vi "op_ACQuisition.vi"(0 "EQ folder path Refnum":refnum<vi>, 1 "HV enable button":bool caption="High Voltage enable", 2 "HV parameters Refnum":refnum<vi>, 3 "HV level Refnum":refnum<vi>, 4 "HV string Refnum":refnum<vi>, 5 "Stop ACQ button Refnum":refnum<vi>, 6 "ACQ Parameters (cluster)":T2={"Acquisition Mode"=0, "Pulse width"=0, "DTP period"=1, "Number of events"=4000} caption="Acquisition Parameters" {"Number of events" min=1; "DTP period" min=1; "Pulse width" items=["25 ns", "50 ns", "75 ns", "100 ns"]; "Acquisition Mode" items=["Normal", "Pedestal", "Test Pulse", "Test Pulse trigger & synchronous"]}, 7 "Events to acquire Refnum":refnum<vi>, 8 "error tick Refnum":refnum<vi>, 9 "ACQ events fets Refnum":refnum<vi>, 10 "Operation text Refnum":refnum<vi>, 11 "ACQ events fets A Refnum":refnum<vi>, 12 "Busy Refnum":refnum<vi>, 13 "ACQ events fets B Refnum":refnum<vi>, 14 "Addresses Cluster":T1={"ENA1"=FALSE, "IP address 1"="172.16.14.22", "ENA2"=FALSE, "IP address 2"="172.16.14.23"}, 15 "etapa# terminals refnums":T3, 17 "GbReg params":u8[](array[numeric])=[32, 22], 19 "Motors Refnum":refnum<vi>) -> (23 "Folder path: acquisition reports":path=path "C:/VIPauto/Files/LayerID/Acquisition/yyyymmdd_hh-mm-ss_Leak#_HV#")   [LabVIEW 2015, in "VIPM2.lvlib"]
uses:
  VIPM2.lvlib
panel:
  out "Chip ID list 2":u32[](array[numeric]) format="%.0x"
  out "Layer ID list 2 (ordered)":u32[](array[numeric]) format="%.0x"
  out "All ID list 2":u32[](array[numeric]) format="%.0x"
  out "All ID list 1":u32[](array[numeric]) format="%.0x"
  out "Layer ID list 1 (ordered)":u32[](array[numeric]) format="%.0x"
  out "Chip ID list 1":u32[](array[numeric]) format="%.0x"
  # "Operation: ACQuisition with HV (refnums)"
  # "Analog Vref low"
  # "Gb THLD"
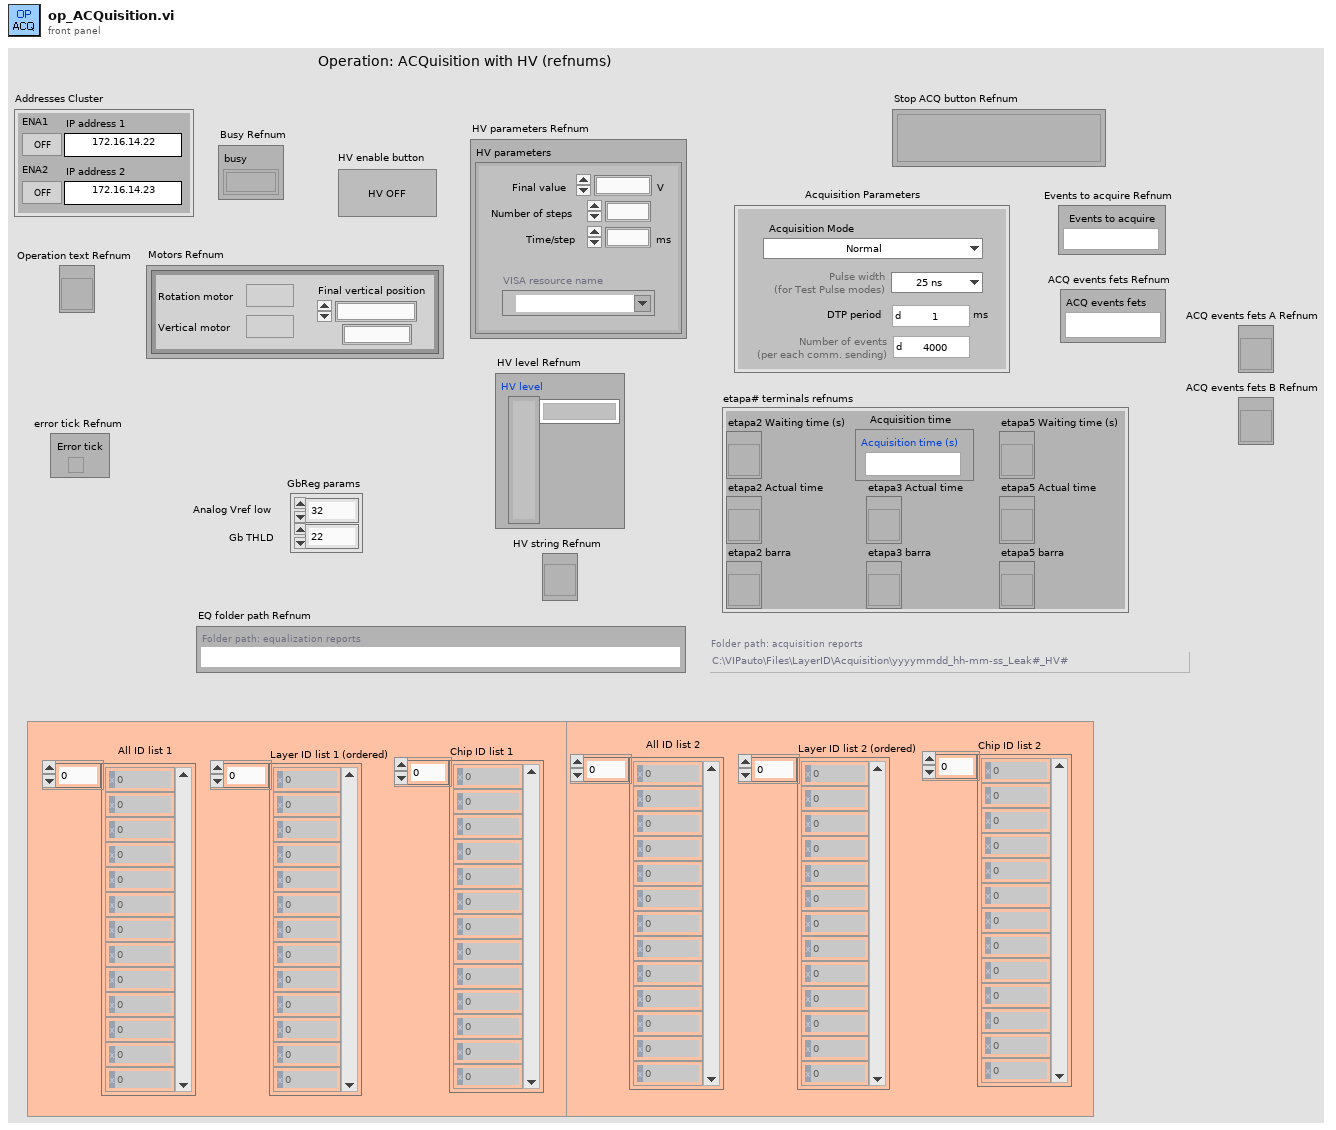
[diagram p1: front panel]
types:
  T1 = cluster{"ENA1":bool, "IP address 1":string, "ENA2":bool, "IP address 2":string}
  T2 = cluster{"Acquisition Mode":u32, "Pulse width":u32, "DTP period":u32, "Number of events":u32}
  T3 = cluster{"etapa2 Waiting time (s)":refnum<vi>, "etapa2 Actual time":refnum<vi>, "etapa2 barra":refnum<vi>, "etapa3 Actual time":refnum<vi>, "etapa3 barra":refnum<vi>, "etapa5 Waiting time (s)":refnum<vi>, "etapa5 Actual time":refnum<vi>, "etapa5 barra":refnum<vi>, "Acquisition time":refnum<vi>}
  T4 = enum8{"Enabled", "Disabled", "Disabled and Grayed Out"}
  T5 = cluster{"Final value":i16, "Number of steps":u8, "Time/step":u16, "Output Off Behavior":u16, "VISA resource name":refnum<visa-resource-name>}
  T6 = cluster{"Rotation motor":bool, "Vertical motor":bool, "Final vertical position":u32, "vertical position":u32}
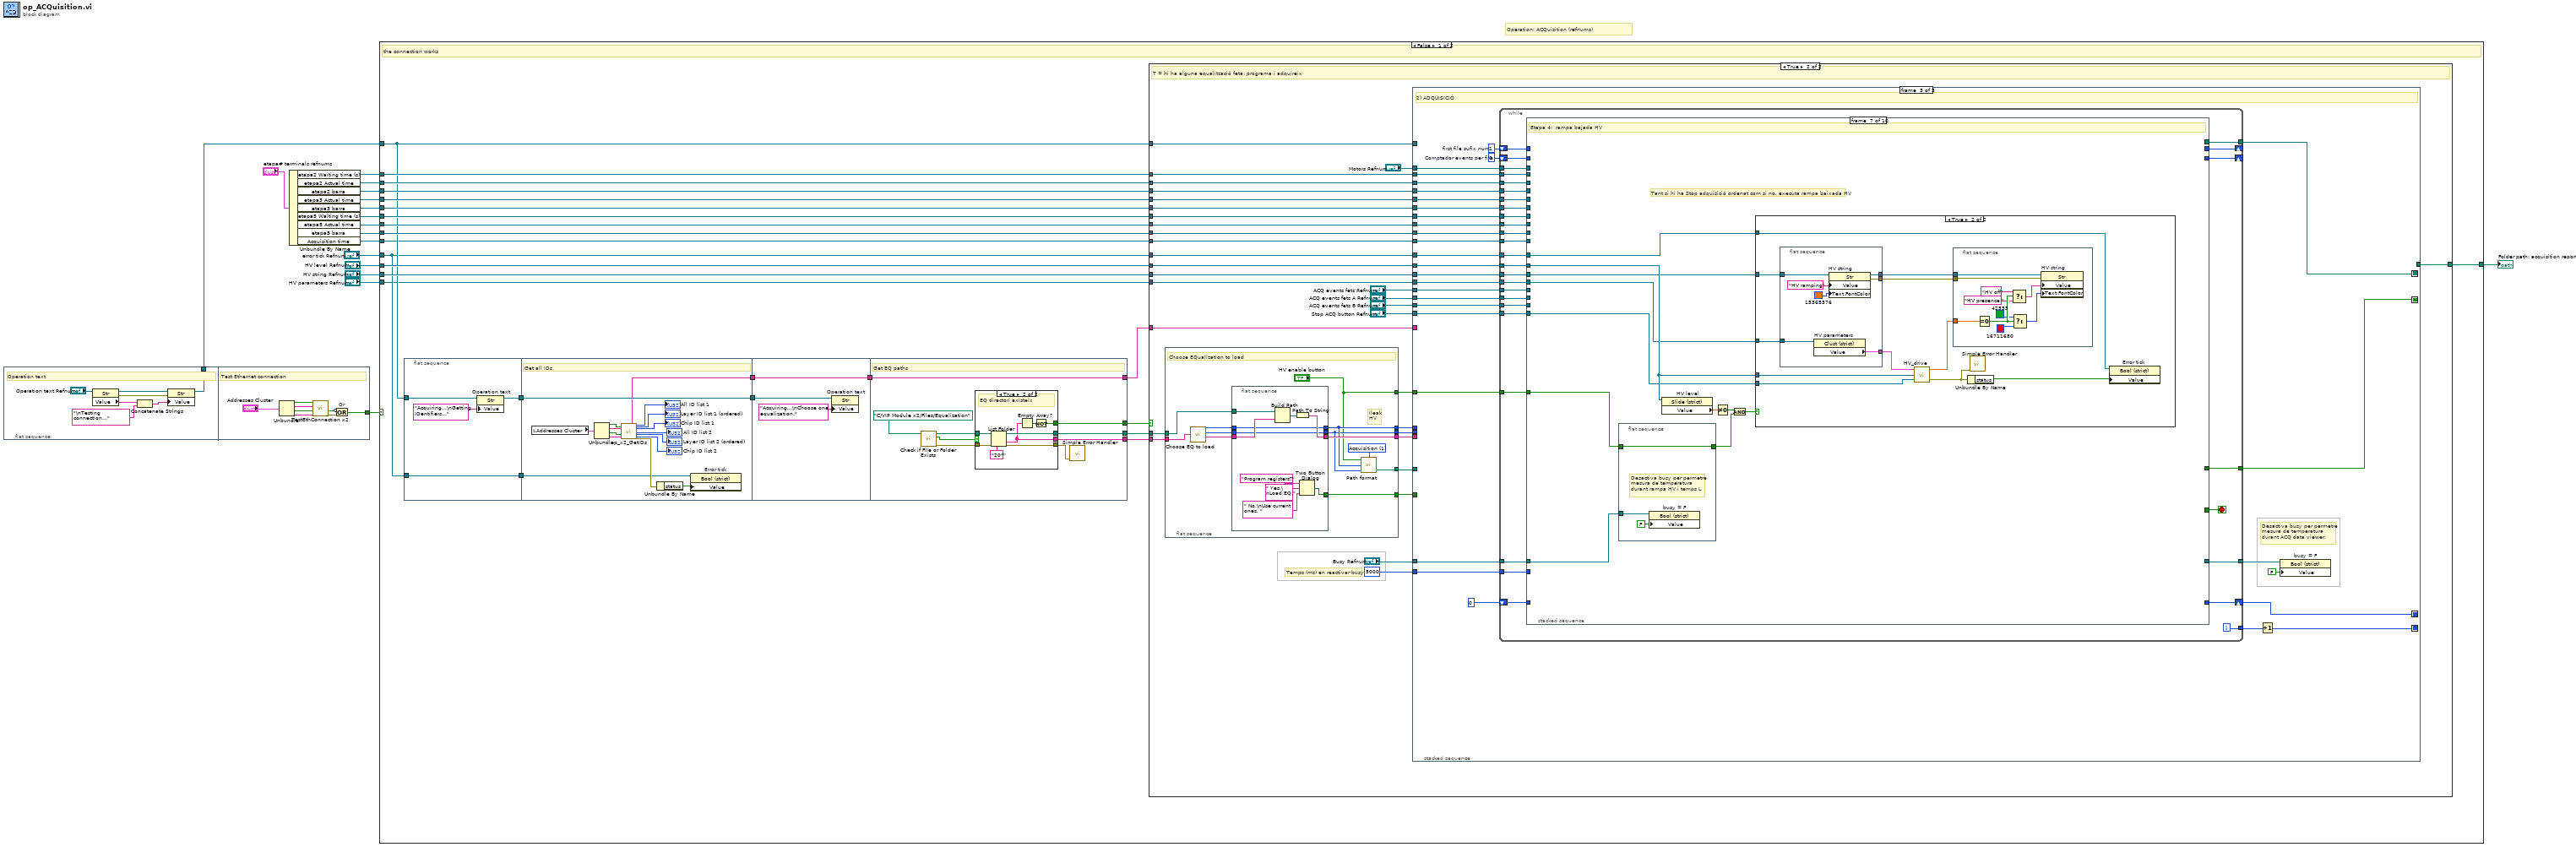
[diagram p0: block diagram]
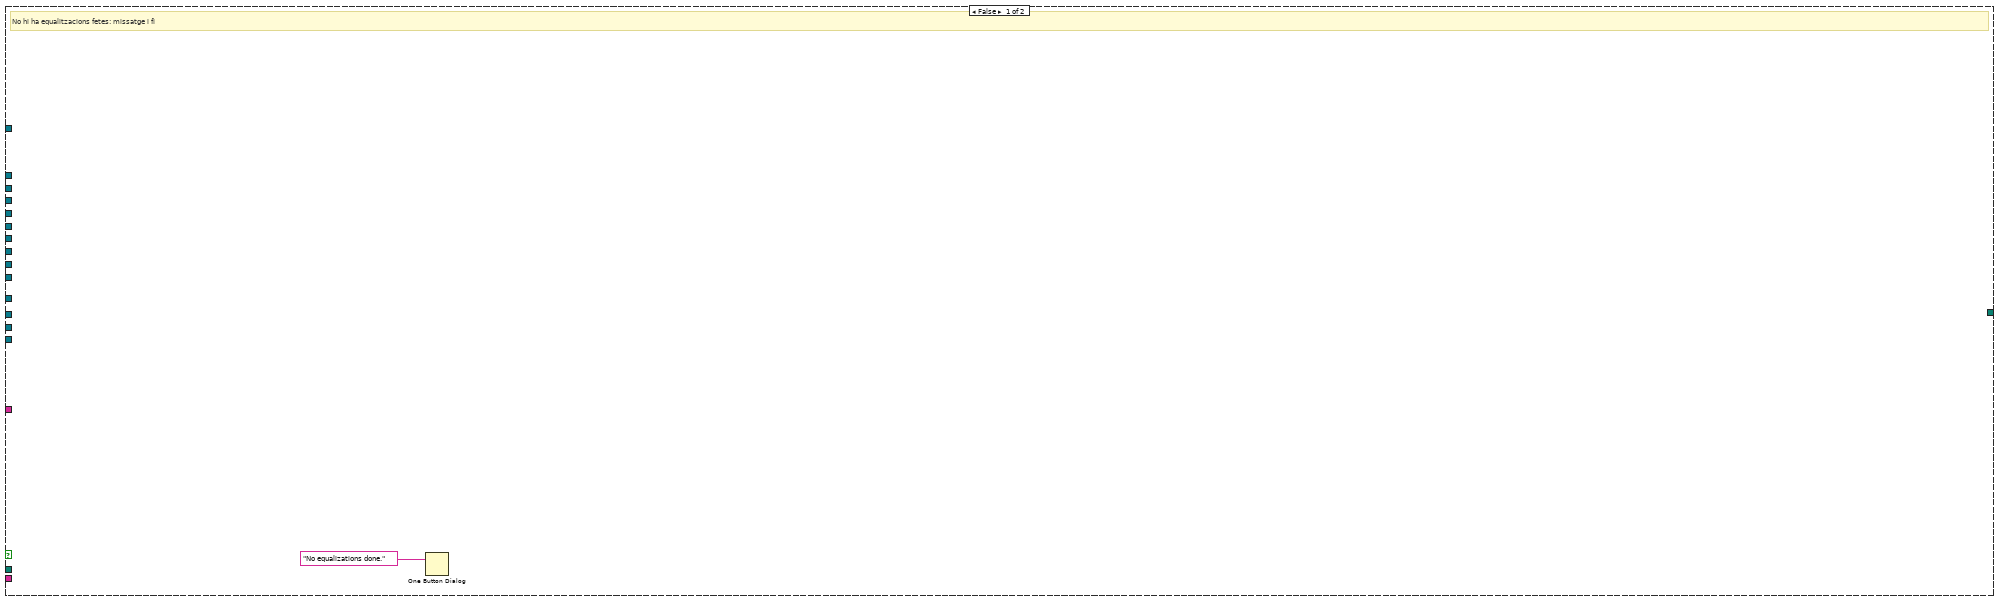
[diagram p3: hidden frame]
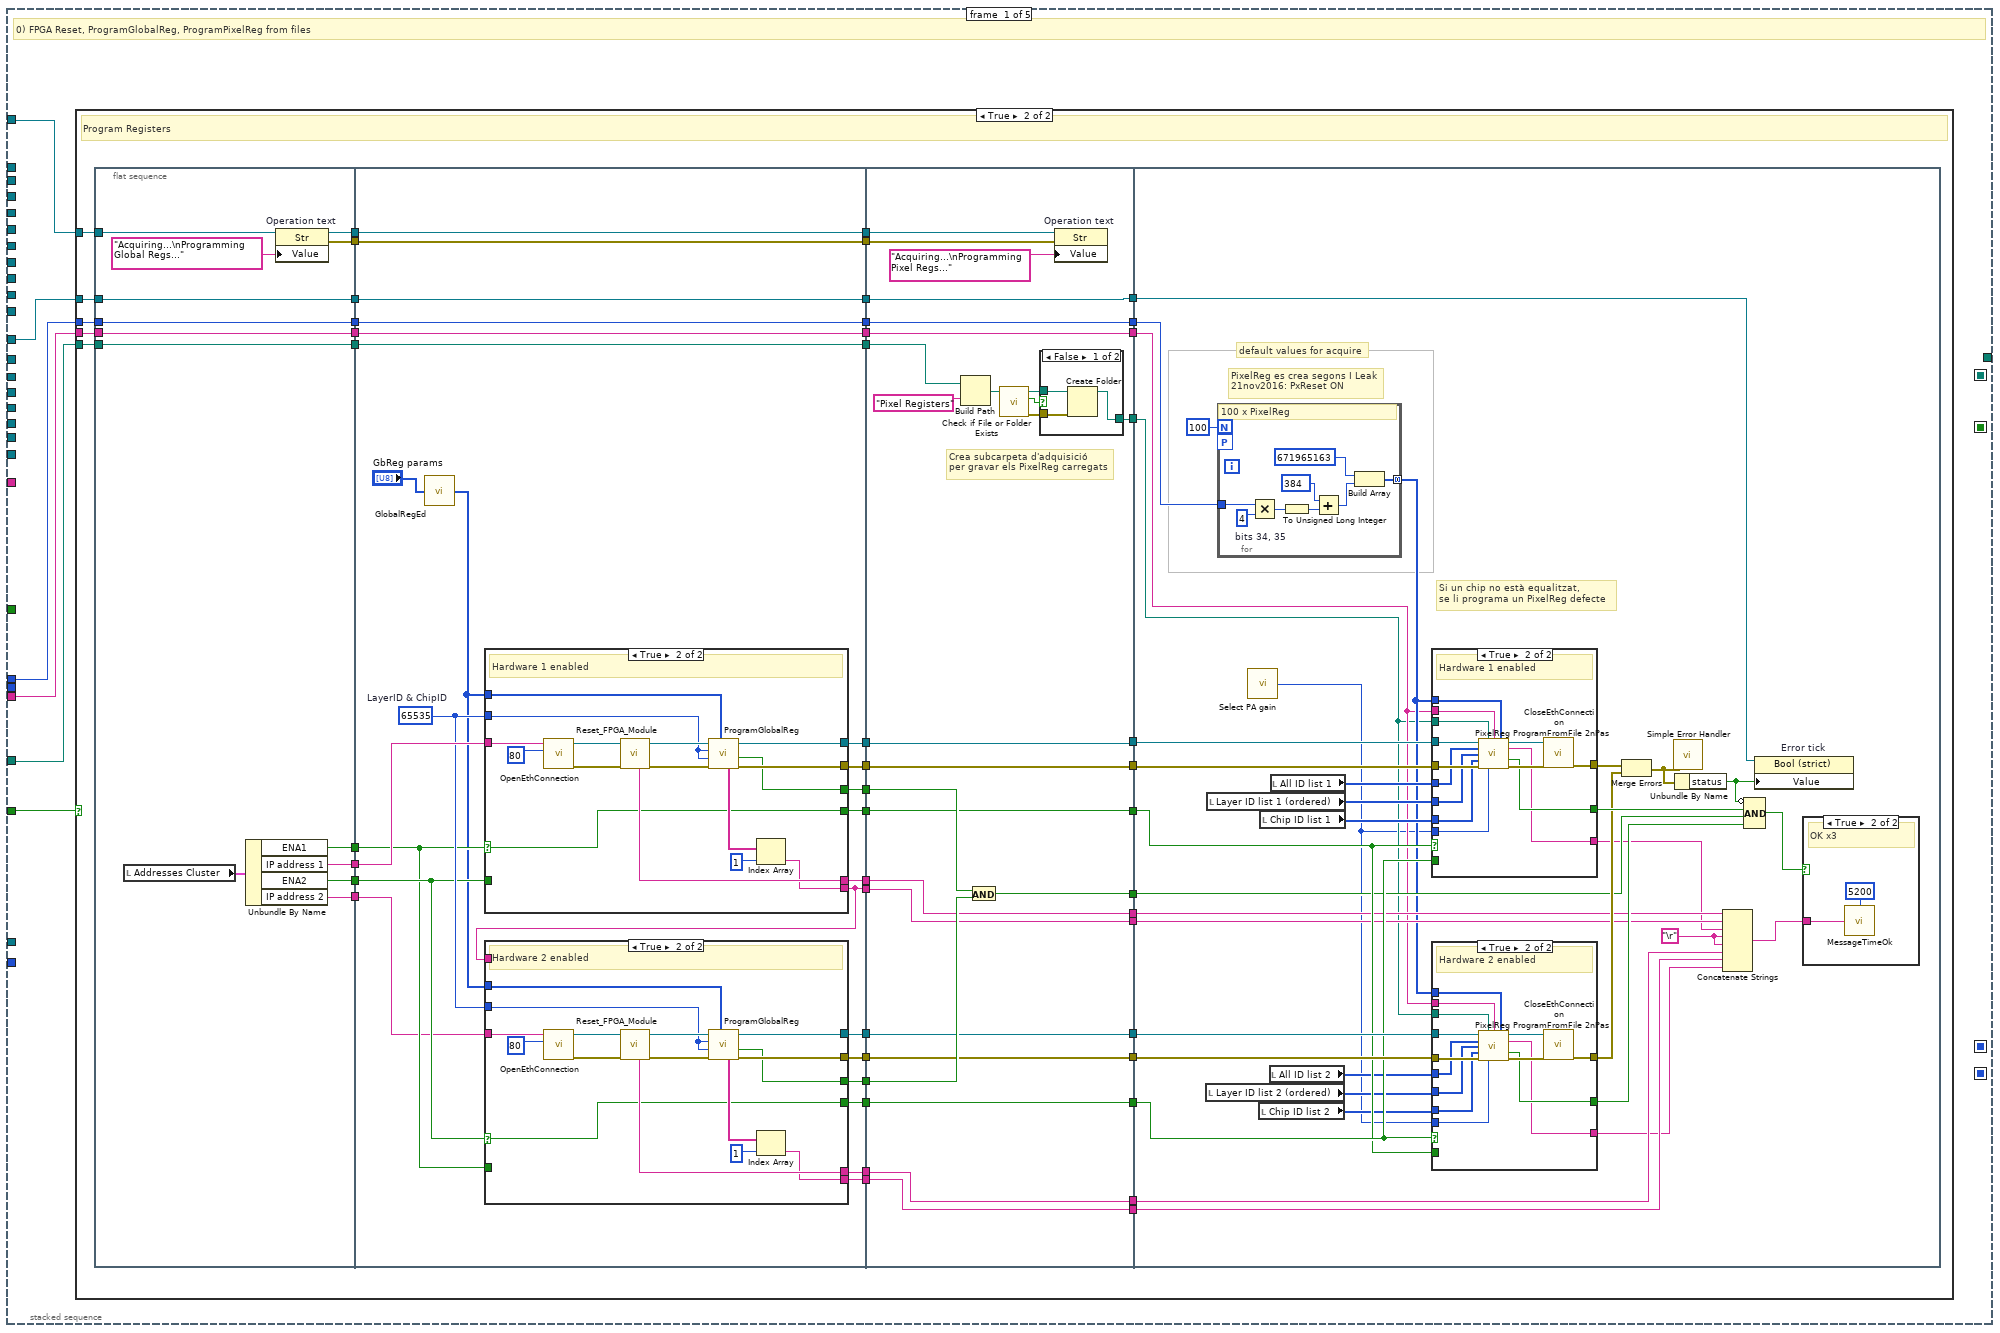
[diagram p4: hidden frame]
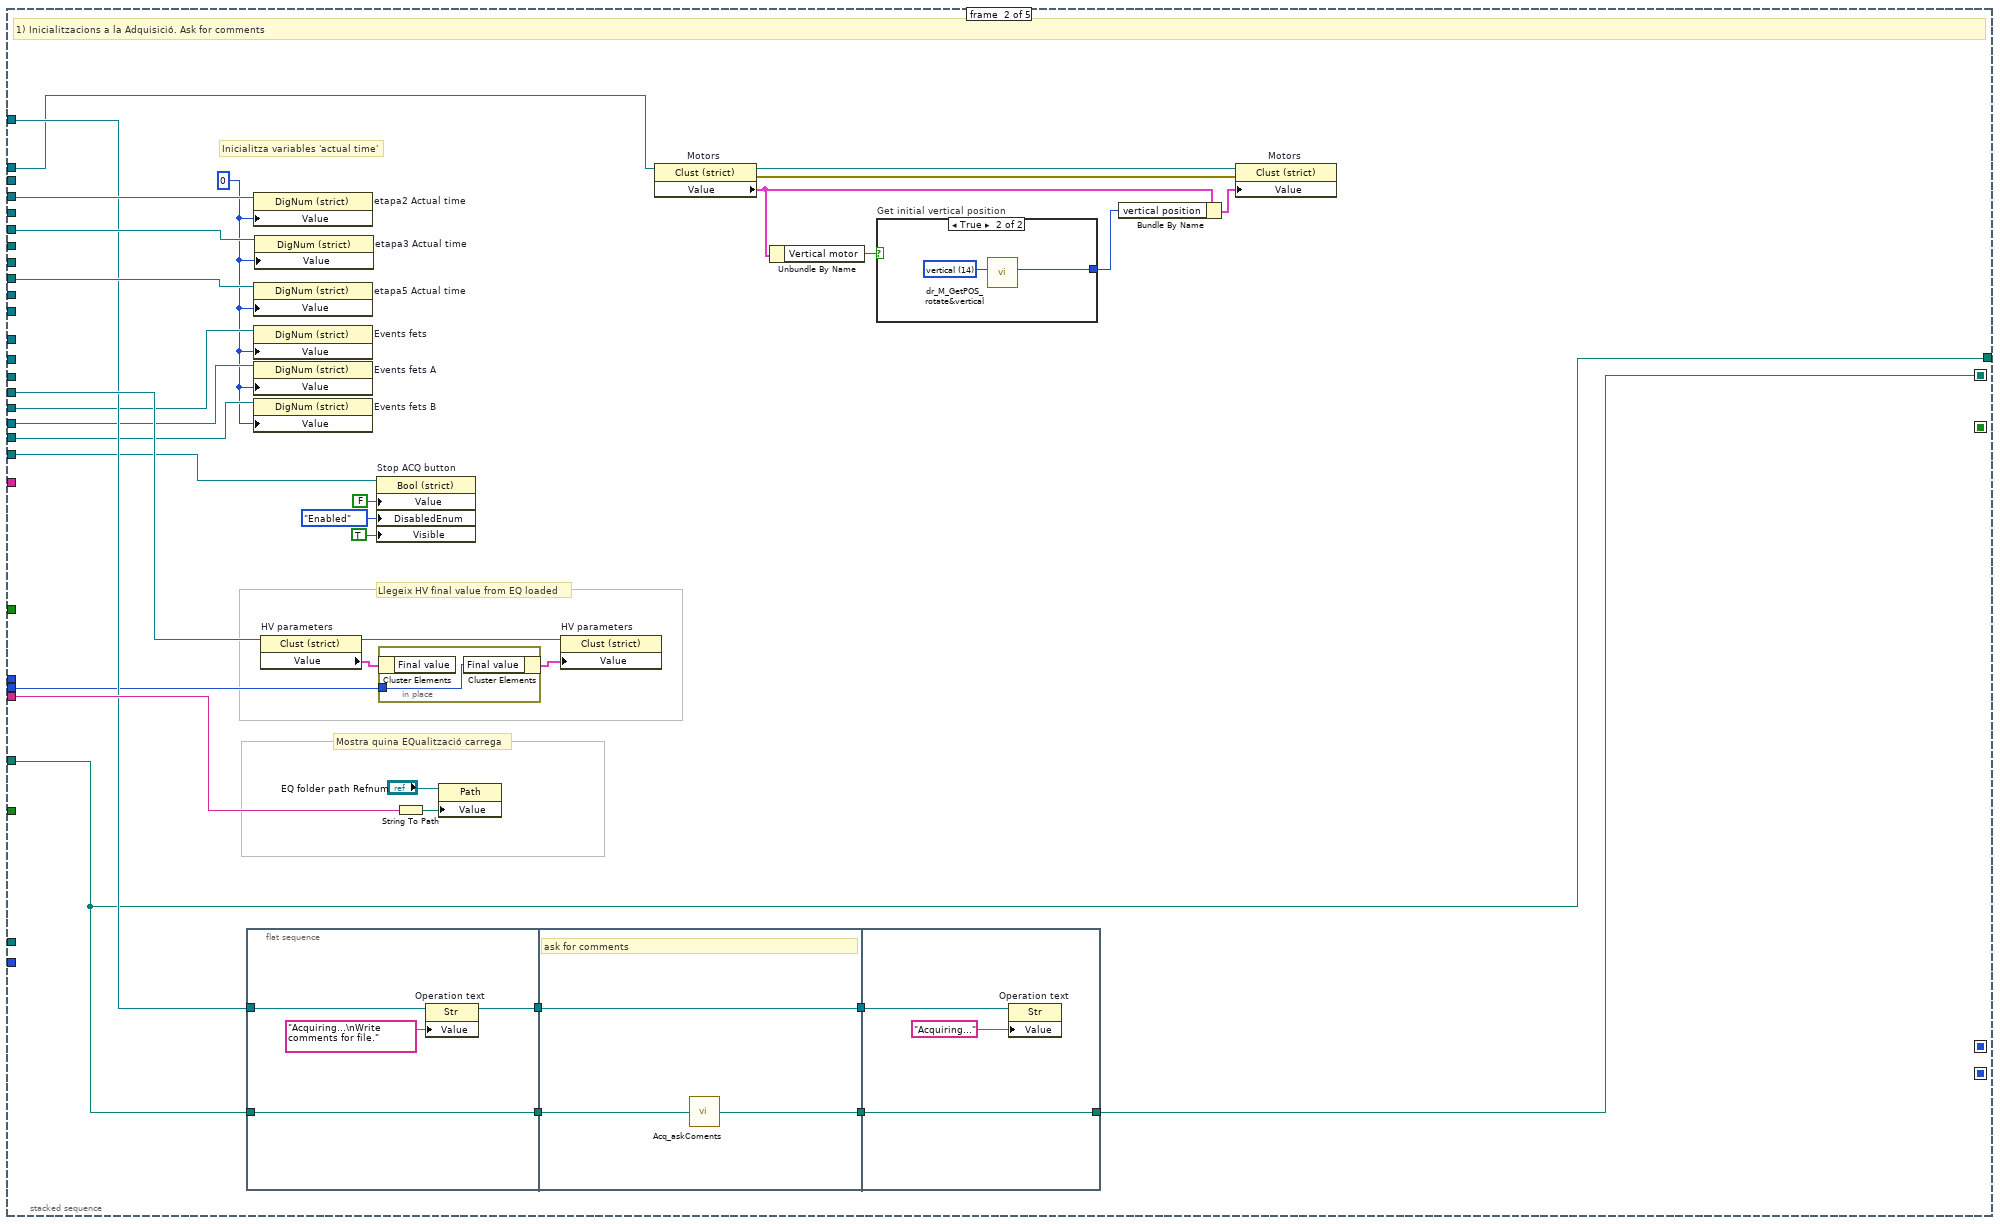
[diagram p12: hidden frame]
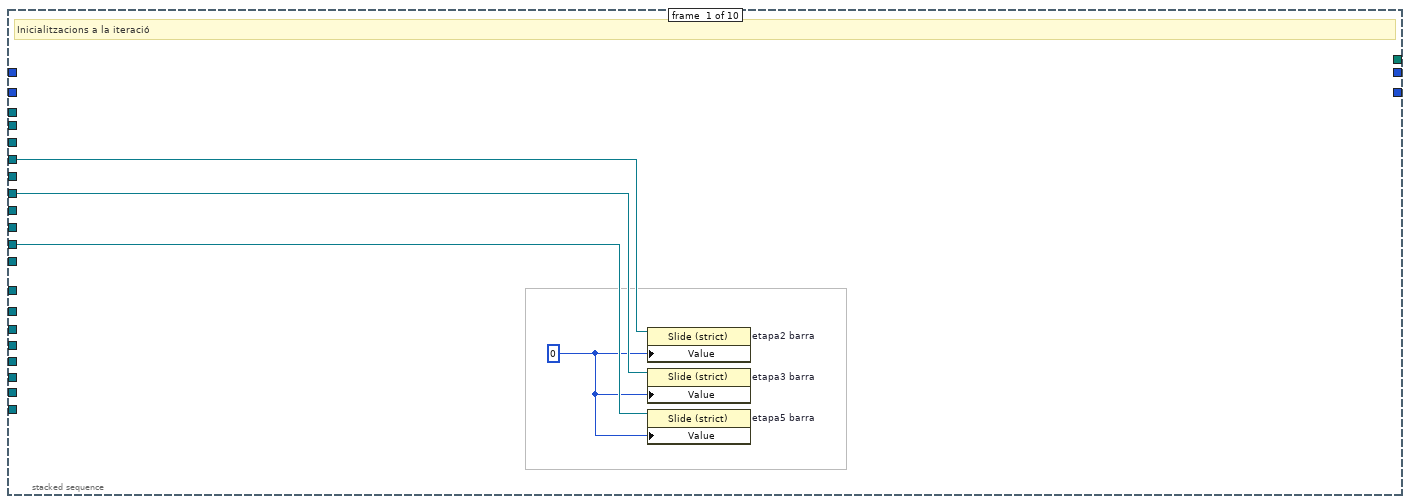
[diagram p14: hidden frame]
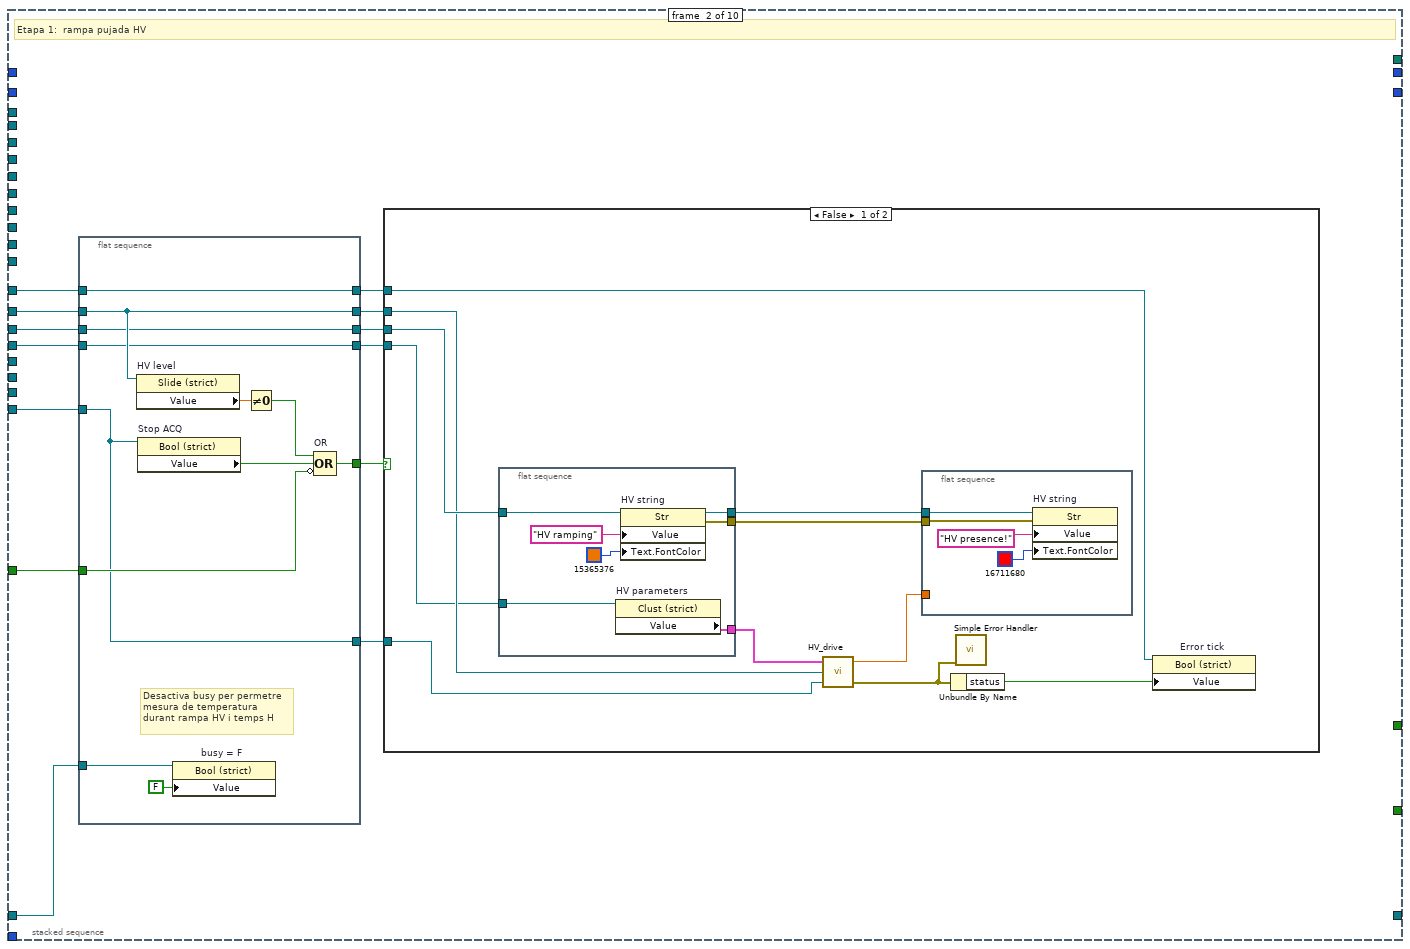
[diagram p15: hidden frame]
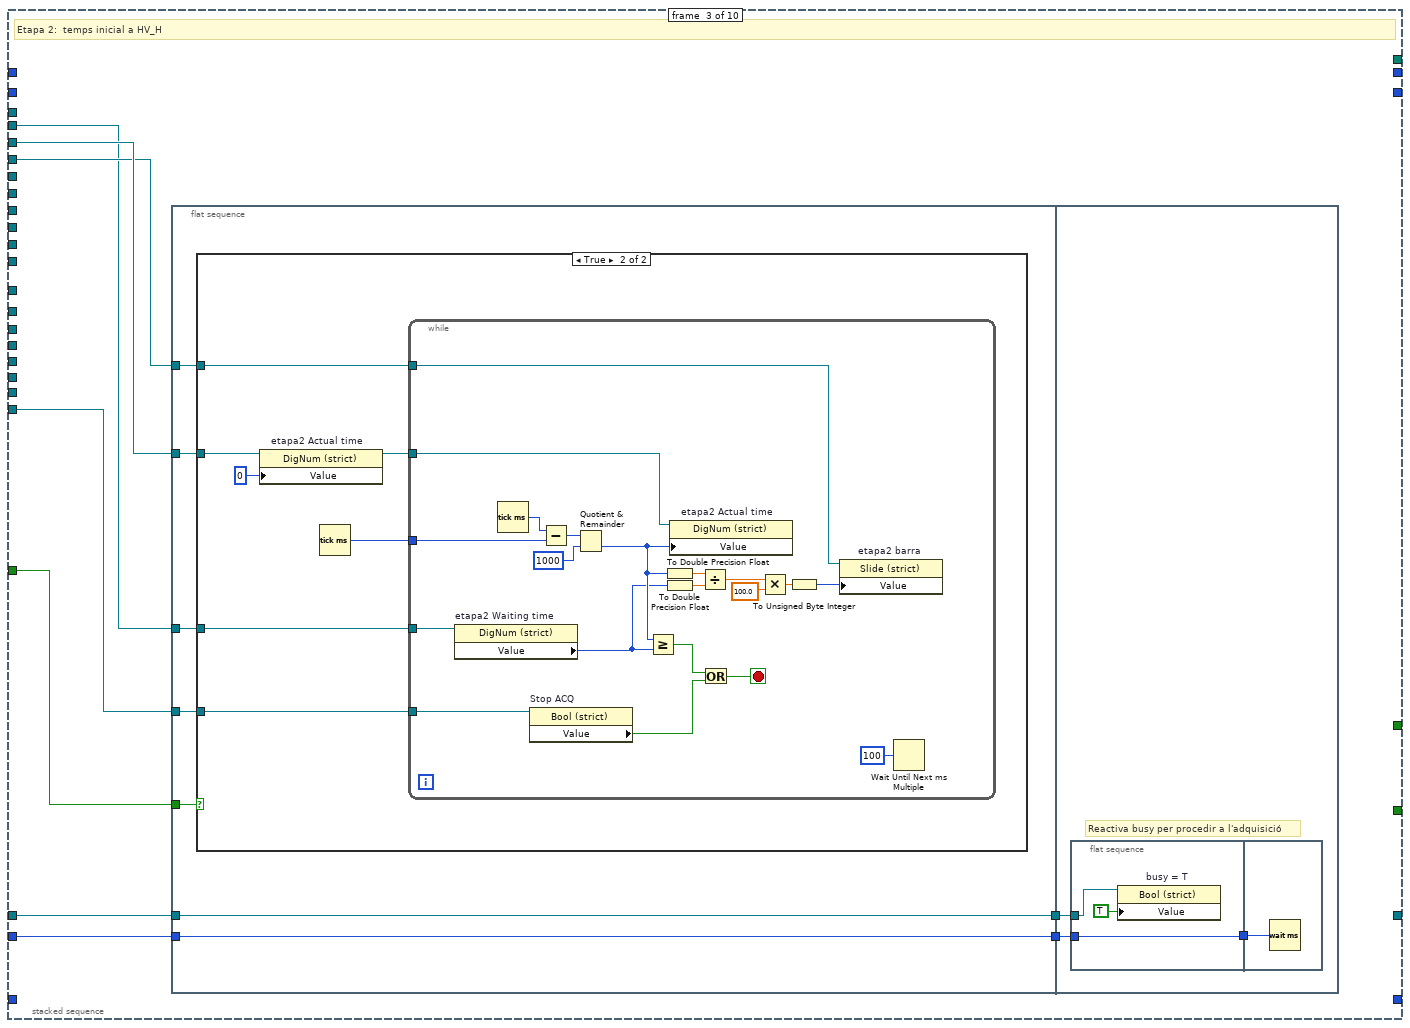
[diagram p17: hidden frame]
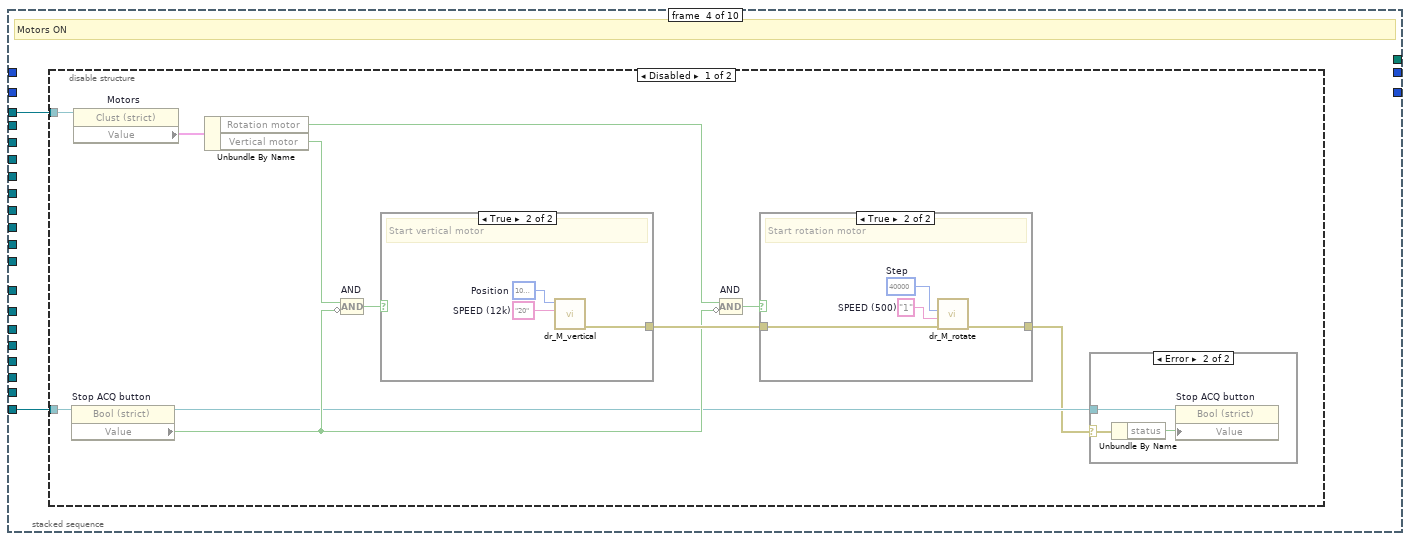
[diagram p19: hidden frame]
diagram:
  # "Operation: ACQuisition (refnums)"
  n1 = flat-sequence {
    tunnel: [w18] -> w7
    tunnel: [w30] -> w17
    frame #0 {
      # "Operation text"
      n2 = property class="Str"(reference="Operation text Refnum") -> (reference out=w21:refnum<vi>, error out=w20:errorcluster, "Value"=w23:string)  [unwired: 1 in]
      n3 = Concatenate Strings "Concatenate Strings"(w23, "\nTesting connection..." ("string")) -> (w19:string)
      n4 = property class="Str"(reference=w21, error in=w20, "Value"=w19) -> (reference out=w18:refnum<vi>)  [unwired: 1 out]
    }
    frame #1 {
      # "Test Ethernet connection"
      n5 = Unbundle("Addresses Cluster") -> ("ENA1"=w28:bool, "IP address 1"=w27:string, "ENA2"=w26:bool, "IP address 2"=w25:string)
      n6 = call "TestEthConnection x2.vi"("IP address 2"=w25, "ENA2"=w26, "IP address 1"=w27, "ENA1"=w28) -> ("error out"=w31:errorcluster, "Answers OK?"=w32:bool)  [unwired: 6 in]
      n7 = Compound Arithmetic op=OR "Or"(invert w32, w31) -> (w30:bool)
    }
  }
  n8 = Unbundle By Name("etapa# terminals refnums") -> ("etapa2 Waiting time (s)"=w15:refnum<vi>, "etapa2 Actual time"=w14:refnum<vi>, "etapa2 barra"=w13:refnum<vi>, "etapa3 Actual time"=w12:refnum<vi>, "etapa3 barra"=w11:refnum<vi>, "etapa5 Waiting time (s)"=w10:refnum<vi>, "etapa5 Actual time"=w9:refnum<vi>, "etapa5 barra"=w8:refnum<vi>, "Acquisition time"=w2:refnum<vi>)
  n9 = case shown="False" w17 {
    selector: w17 -> [_ w939]
    tunnel: w15 -> [w56 _]
    tunnel: w14 -> [w55 _]
    tunnel: w13 -> [w54 _]
    tunnel: w12 -> [w53 _]
    tunnel: w11 -> [w52 _]
    tunnel: w10 -> [w51 _]
    tunnel: w9 -> [w50 _]
    tunnel: w8 -> [w49 _]
    tunnel: w7 -> [w45 _]
    tunnel: "HV level Refnum" -> [w48 _]
    tunnel: "HV string Refnum" -> [w47 _]
    tunnel: "error tick Refnum" -> [w43 w938]
    tunnel: [w46 _] -> w1
    tunnel: "HV parameters Refnum" -> [w37 _]
    tunnel: w2 -> [w36 _]
    frame False {
      # "the connection works"
      n10 = flat-sequence {
        tunnel: w45 -> [w60]
        tunnel: [w58] -> w44
        tunnel: w43 -> [w58]
        tunnel: [w57] -> w41
        tunnel: w44 -> [w74]
        tunnel: [w73] -> w42
        tunnel: w41 -> [w73]
        tunnel: [w72] -> w34
        tunnel: w42 -> [w78]
        tunnel: [w77] -> w35
        tunnel: w34 -> [w77]
        tunnel: [w84] -> w40
        tunnel: [w83] -> w39
        tunnel: [w82] -> w38
        tunnel: [w80] -> w33
        tunnel: w35 -> [w80]
        frame #0 {
          n11 = property on="Operation text" class="Str"(reference=w60, "Value"="Acquiring...\nGetting IDentifiers...") -> (reference out=w57:refnum<vi>)  [unwired: 1 in, 1 out]
        }
        frame #1 {
          # "Get all IDs"
          n12 = local read "Addresses Cluster"() -> (w71:T1)
          n13 = Unbundle(w71) -> ("ENA1"=w70:bool, "IP address 1"=w69:string, "ENA2"=w67:bool, "IP address 2"=w68:string)
          n14 = call "op_x2_GetIDs.vi"("ENA1"=w70, "IP address 1"=w69, "ENA2"=w67, "IP address 2"=w68) -> ("summary IDs"=w72:string, "All ID list 1"=→"All ID list 1":u32[], "Layer ID list 1 (ordered)"=→"Layer ID list 1 (ordered)":u32[], "Chip ID list 1"=→"Chip ID list 1":u32[], "All ID list 2"=→"All ID list 2":u32[], "Layer ID list 2 (ordered)"=→"Layer ID list 2 (ordered)":u32[], "Chip ID list 2"=→"Chip ID list 2":u32[], "error out"=w75:errorcluster)  [unwired: 16 in]
          n15 = Unbundle By Name(w75) -> ("status"=w76:bool)
          n16 = property on="Error tick" class="Bool (strict)"(reference=w74, "Value"=w76) -> ()  [unwired: 1 in, 2 out]
        }
        frame #2 {
          n17 = property on="Operation text" class="Str"(reference=w78, "Value"="Acquiring...\nChoose one equalization.") -> ()  [unwired: 1 in, 2 out]
        }
        frame #3 {
          # "Get EQ paths"
          n18 = call <vilib>:"Check if File or Folder Exists.vi"("path"=path "C:/VIP Module x2/Files/Equalization") -> ("error out"=w85:errorcluster, "file or folder exists?"=w86:bool, "dup path"=w87:path)  [unwired: 8 in]
          n19 = case shown="True" w86 {
            selector: w86 -> [w91 _]
            tunnel: w87 -> [w90 w97]
            tunnel: w85 -> [w89 w96]
            tunnel: [w91 w93] -> w84
            tunnel: [w90 w94] -> w83
            tunnel: [w89 w95] -> w81
            tunnel: [_ w92] -> w82
            frame False {
              # "no EQs"
            }
            frame True {
              # "EQ directori existeix"
              n20 = List Folder(path=w97, pattern="20*", error in=w96) -> (path out=w94:path, folder names=w92:string[], error out=w95:errorcluster)  [unwired: 1 in, 1 out]
              n21 = Empty Array?(array=w92) -> (empty?=w98:bool)
              n22 = Not(x=w98) -> (.not. x?=w93:bool)
            }
          }
          n23 = call <vilib>:"Simple Error Handler.vi"("error in (no error)"=w81) -> ()  [unwired: 4 in, 5 out]
        }
      }
      n24 = case shown="True" w40 {
        tunnel: w56 -> [_ w131]
        tunnel: w55 -> [_ w130]
        tunnel: w54 -> [_ w129]
        tunnel: w53 -> [_ w128]
        tunnel: w52 -> [_ w127]
        tunnel: w51 -> [_ w126]
        tunnel: w50 -> [_ w125]
        tunnel: w49 -> [_ w124]
        tunnel: w48 -> [_ w123]
        tunnel: w47 -> [_ w122]
        tunnel: [_ w121] -> w46
        tunnel: w45 -> [_ w120]
        tunnel: w43 -> [_ w119]
        tunnel: w39 -> [_ w118]
        tunnel: w38 -> [_ w117]
        tunnel: w37 -> [_ w113]
        tunnel: w36 -> [_ w110]
        tunnel: w33 -> [_ w108]
        frame False {
          # "No hi ha equalitzacions fetes: missatge i fi"
          n25 = One Button Dialog(message="No equalizations done.") -> ()  [unwired: 1 in, 1 out]
        }
        frame True {
          # "Temps (ms) en reactivar busy"
          # "T = hi ha alguna equalització feta: programa i adquireix"
          n26 = flat-sequence {
            tunnel: w118 -> [w140]
            tunnel: w117 -> [w141]
            tunnel: [w138] -> w116
            tunnel: [w133] -> w115
            tunnel: [w136] -> w114
            tunnel: [w142] -> w112
            tunnel: [w137] -> w107
            tunnel: ["HV enable button"] -> w104
            frame #0 {
              w143 = u8 1 items=["Equalization", "Acquisition"] ("Operation type")
              # "Ileak\nHV"
              # "Choose EQualization to load"
              n27 = call "Choose EQ to load.vi"("EQ folders"=w141) -> ("I Leakage"=w135:u8, "HV last value"=w134:i16, "loaded EQ folder"=w139:string)  [unwired: 5 in]
              n28 = flat-sequence {
                tunnel: w140 -> [w153]
                tunnel: w139 -> [w152]
                tunnel: [w150] -> w138
                tunnel: [w149] -> w137
                tunnel: [w145] -> w136
                tunnel: w135 -> [w145]
                tunnel: w134 -> [w144]
                tunnel: [w144] -> w133
                frame #0 {
                  n29 = Build Path(base path=w153, name or relative path=w152) -> (appended path=w151:path)
                  n30 = Path To String(path=w151) -> (string=w150:string)
                  n31 = Two Button Dialog(message="Program registers?", 1:" No.\nUse current ones. " ("F button name (\"Cancel\")"), 2:" Yes.\nLoad EQ." ("T button name (\"OK\")")) -> (T button?=w149:bool)
                }
              }
              n32 = call "Path format.vi"("Operation type"=w143, "HV level"=w133, "I leakage"=w136, "HV enable button"="HV enable button") -> ("folder path"=w142:path)  [unwired: 1 in]
            }
          }
          n33 = stacked-sequence {
            seq-local: [_ _ w450 _ _] -> [_ _ _ _ w890]
            seq-local: [_ w406 _ _ _] -> [_ _ w451 _ w889]
            seq-local: [_ _ w441 _ _] -> [_ _ _ _ w868]
            seq-local: [_ _ w439 _ _] -> [_ _ _ _ w867]
            tunnel: w120 -> [w159 w411 _ _ w887]
            tunnel: w131 -> [_ _ w465 _ w874]
            tunnel: w130 -> [_ w421 w464 _ _]
            tunnel: w129 -> [_ _ w463 _ _]
            tunnel: w128 -> [_ w420 w462 _ _]
            tunnel: w127 -> [_ _ w461 _ _]
            tunnel: w126 -> [_ _ w460 _ w876]
            tunnel: w125 -> [_ w419 w459 _ _]
            tunnel: w124 -> [_ _ w458 _ _]
            tunnel: w119 -> [w158 _ w455 _ _]
            tunnel: w123 -> [_ _ w457 _ _]
            tunnel: w122 -> [_ _ w456 _ _]
            tunnel: [_ w404 _ _ _] -> w121
            tunnel: w116 -> [w157 w412 _ _ w881]
            tunnel: w115 -> [_ w410 _ _ _]
            tunnel: w114 -> [w156 _ _ _ _]
            tunnel: w113 -> [_ w418 w454 _ w885]
            tunnel: w112 -> [w155 w404 _ _ w882]
            tunnel: "Stop ACQ button Refnum" -> [_ w403 w453 w866 _]
            tunnel: w110 -> [_ _ w452 _ w875]
            tunnel: "ACQ events fets Refnum" -> [_ w399 w449 _ w880]
            tunnel: w108 -> [_ _ _ _ w888]
            tunnel: w107 -> [w154 _ _ _ w883]
            tunnel: "Busy Refnum" -> [_ _ w448 _ _]
            tunnel: u32 5000 -> [_ _ w447 _ _]
            tunnel: w104 -> [_ _ w443 _ _]
            tunnel: "ACQ events fets A Refnum" -> [_ w398 w438 _ _]
            tunnel: "ACQ events fets B Refnum" -> [_ w397 w437 _ _]
            tunnel: "Motors Refnum" -> [_ w395 w435 _ _]
            frame #0 {
              # "0) FPGA Reset, ProgramGlobalReg, ProgramPixelReg from files"
              n34 = case shown="True" w154 {
                tunnel: w159 -> [_ w190]
                tunnel: w158 -> [_ w189]
                tunnel: w157 -> [_ w188]
                tunnel: w156 -> [_ w187]
                tunnel: w155 -> [_ w186]
                frame False {
                  # "Use current registers values"
                }
                frame True {
                  # "Program Registers"
                  n35 = flat-sequence {
                    tunnel: w190 -> [w219]
                    tunnel: [w218] -> w207
                    tunnel: [w217] -> w206
                    tunnel: [w216] -> w205
                    tunnel: w189 -> [w216]
                    tunnel: [w215] -> w204
                    tunnel: w188 -> [w215]
                    tunnel: [w214] -> w203
                    tunnel: w187 -> [w214]
                    tunnel: [w213] -> w202
                    tunnel: w186 -> [w213]
                    tunnel: [w211] -> w185
                    tunnel: [w210] -> w184
                    tunnel: [w209] -> w183
                    tunnel: [w208] -> w182
                    tunnel: w207 -> [w245]
                    tunnel: w206 -> [w244]
                    tunnel: [w245] -> w201
                    tunnel: [w244] -> w200
                    tunnel: [w243] -> w199
                    tunnel: w205 -> [w243]
                    tunnel: w204 -> [w242]
                    tunnel: [w242] -> w198
                    tunnel: w203 -> [w241]
                    tunnel: [w241] -> w197
                    tunnel: w202 -> [w240]
                    tunnel: [w240] -> w196
                    tunnel: w185 -> [w236]
                    tunnel: w184 -> [w237]
                    tunnel: w183 -> [w239]
                    tunnel: w182 -> [w235]
                    tunnel: [w234] -> w181
                    tunnel: [w233] -> w180
                    tunnel: [w232] -> w179
                    tunnel: [w231] -> w178
                    tunnel: [w230] -> w177
                    tunnel: [w223] -> w176
                    tunnel: [w229] -> w175
                    tunnel: [w228] -> w174
                    tunnel: [w227] -> w173
                    tunnel: [w226] -> w172
                    tunnel: [w225] -> w171
                    tunnel: [w224] -> w170
                    tunnel: w201 -> [w306]
                    tunnel: w200 -> [w305]
                    tunnel: [w292] -> w195
                    tunnel: [w291] -> w194
                    tunnel: [w304] -> w193
                    tunnel: w199 -> [w304]
                    tunnel: [w303] -> w192
                    tunnel: w198 -> [w303]
                    tunnel: [w302] -> w191
                    tunnel: w197 -> [w302]
                    tunnel: w196 -> [w294]
                    tunnel: w181 -> [w292]
                    tunnel: w180 -> [w291]
                    tunnel: w179 -> [w301]
                    tunnel: w178 -> [w290]
                    tunnel: w177 -> [w285]
                    tunnel: w176 -> [w284]
                    tunnel: w175 -> [w289]
                    tunnel: w174 -> [w288]
                    tunnel: w173 -> [w300]
                    tunnel: w172 -> [w287]
                    tunnel: w171 -> [w283]
                    tunnel: w170 -> [w282]
                    tunnel: [w293] -> w169
                    tunnel: [w290] -> w168
                    tunnel: [w289] -> w167
                    tunnel: [w288] -> w166
                    tunnel: [w287] -> w165
                    tunnel: [w286] -> w164
                    tunnel: [w285] -> w163
                    tunnel: [w284] -> w162
                    tunnel: [w283] -> w161
                    tunnel: [w282] -> w160
                    tunnel: w195 -> [w341]
                    tunnel: w194 -> [w340]
                    tunnel: w193 -> [w343]
                    tunnel: w192 -> [w319]
                    tunnel: w191 -> [w338]
                    tunnel: w169 -> [w318]
                    tunnel: w168 -> [w331]
                    tunnel: w167 -> [w334]
                    tunnel: w166 -> [w333]
                    tunnel: w165 -> [w332]
                    tunnel: w164 -> [w324]
                    tunnel: w163 -> [w322]
                    tunnel: w162 -> [w321]
                    tunnel: w161 -> [w315]
                    tunnel: w160 -> [w314]
                    frame #0 {
                      n36 = local read "Addresses Cluster"() -> (w212:T1)
                      n37 = Unbundle By Name(w212) -> ("ENA1"=w211:bool, "IP address 1"=w209:string, "ENA2"=w210:bool, "IP address 2"=w208:string)
                      n38 = property on="Operation text" class="Str"(reference=w219, "Value"="Acquiring...\nProgramming Global Regs...") -> (reference out=w218:refnum<vi>, error out=w217:errorcluster)  [unwired: 1 in]
                    }
                    frame #1 {
                      w238 = u32 65535  # LayerID & ChipID
                      n39 = call "GlobalRegEd.vi"("params"="GbReg params") -> ("Global Reg out"=w222:u32[])  [unwired: 4 in]
                      n40 = case shown="True" w236 {
                        selector: w236 -> [w265 w266]
                        tunnel: w238 -> [_ w268]
                        tunnel: [_ w274] -> w234
                        tunnel: [_ w273] -> w233
                        tunnel: [_ w272] -> w230
                        tunnel: [_ w271] -> w223
                        tunnel: [w264 w270] -> w232
                        tunnel: w222 -> [_ w269]
                        tunnel: w239 -> [_ w267]
                        tunnel: [w265 w266] -> w231
                        tunnel: w237 -> [w264 _]
                        frame False {
                          # "Hardware 1 not enabled"
                        }
                        frame True {
                          # "Hardware 1 enabled"
                          n41 = call "OpenEthConnection.vi"("Port"=u16 80, "IP address"=w267) -> ("error out"=w280:errorcluster, "connection ID out"=w281:refnum<k5>)  [unwired: 7 in, 1 out]
                          n42 = call "Reset_FPGA_Module.vi"("error in (no error)"=w280, "connection ID"=w281) -> ("error out"=w277:errorcluster, "connection ID out"=w278:refnum<k5>, "Answer to Reset"=w272:string)  [unwired: 7 in]
                          n43 = call "ProgramGlobalReg.vi"("Global Reg"=w269, "error in (no error)"=w277, "ChipID"=w268, "LayerID"=w268, "connection ID"=w278) -> ("error out"=w273:errorcluster, "OK?"=w270:bool, "connection ID out"=w274:refnum<k5>, "Program done"=w276:string[])  [unwired: 2 in, 1 out]
                          n44 = Index Array "Index Array"(array=w276, index=1) -> (element=w271:string)
                        }
                      }
                      n45 = case shown="True" w237 {
                        selector: w237 -> [w247 w248]
                        tunnel: w238 -> [_ w250]
                        tunnel: [_ w256] -> w229
                        tunnel: [_ w255] -> w228
                        tunnel: [_ w254] -> w225
                        tunnel: [_ w253] -> w224
                        tunnel: [w246 w252] -> w227
                        tunnel: w222 -> [_ w251]
                        tunnel: w235 -> [_ w249]
                        tunnel: [w247 w248] -> w226
                        tunnel: w236 -> [w246 _]
                        tunnel: w223 -> [_ _]
                        frame False {
                          # "Hardware 2 not enabled"
                        }
                        frame True {
                          # "Hardware 2 enabled"
                          n46 = call "OpenEthConnection.vi"("Port"=u16 80, "IP address"=w249) -> ("error out"=w262:errorcluster, "connection ID out"=w263:refnum<k5>)  [unwired: 7 in, 1 out]
                          n47 = call "Reset_FPGA_Module.vi"("error in (no error)"=w262, "connection ID"=w263) -> ("error out"=w259:errorcluster, "connection ID out"=w260:refnum<k5>, "Answer to Reset"=w254:string)  [unwired: 7 in]
                          n48 = call "ProgramGlobalReg.vi"("Global Reg"=w251, "error in (no error)"=w259, "ChipID"=w250, "LayerID"=w250, "connection ID"=w260) -> ("error out"=w255:errorcluster, "OK?"=w252:bool, "connection ID out"=w256:refnum<k5>, "Program done"=w258:string[])  [unwired: 2 in, 1 out]
                          n49 = Index Array "Index Array"(array=w258, index=1) -> (element=w253:string)
                        }
                      }
                    }
                    frame #2 {
                      # "Crea subcarpeta d'adquisició\nper gravar els PixelReg carregats"
                      n50 = Build Path(base path=w294, name or relative path="Pixel Registers") -> (appended path=w298:path)
                      n51 = And(x=w301, y=w300) -> (x .and. y?=w286:bool)
                      n52 = call <vilib>:"Check if File or Folder Exists.vi"("path"=w298) -> ("error out"=w295:errorcluster, "file or folder exists?"=w297:bool, "dup path"=w296:path)  [unwired: 8 in]
                      n53 = case shown="False" w297 {
                        tunnel: w296 -> [w310 w311]
                        tunnel: w295 -> [w309 _]
                        tunnel: [w308 w311] -> w293
                        frame False {
                          n54 = Create Folder(path (use dialog)=w310, error in=w309) -> (created path=w308:path)  [unwired: 1 in, 2 out]
                        }
                        frame True {
                        }
                      }
                      n55 = property on="Operation text" class="Str"(reference=w306, error in=w305, "Value"="Acquiring...\nProgramming Pixel Regs...") -> ()  [unwired: 2 out]
                    }
                    frame #3 {
                      w316 = "\r"
                      # "Si un chip no està equalitzat,\nse li programa un PixelReg defecte"
                      # "default values for acquire"
                      # "PixelReg es crea segons I Leak\n21nov2016: PxReset ON"
                      n56 = local read "Layer ID list 2 (ordered)"() -> (w329:u32[])
                      n57 = local read "Layer ID list 1 (ordered)"() -> (w336:u32[])
                      n58 = for {
                        N: 100 -> [_]
                        tunnel: w338 -> [w382]
                        tunnel: [w379] -> w320 mode=concatenating
                        workers-P: _ -> [_]
                        w386 = u8 4  # bits 34, 35
                        # "100 x PixelReg"
                        n59 = Multiply(x=w382, y=w386) -> (x*y=w384:u8)
                        n60 = To Unsigned Long Integer(number=w384) -> (unsigned 32bit integer=w383:u32)
                        n61 = Add(x=u32 384, y=w383) -> (x+y=w380:u32)
                        n62 = Build Array(u32 671965163 ("Numeric"), w380) -> (w379:u32[])
                      }
                      n63 = call "Select PA gain.vi"() -> ("PA gain selected"=w312:u8)  [unwired: 5 in]
                      n64 = local read "Chip ID list 2"() -> (w328:u32[])
                      n65 = local read "Chip ID list 1"() -> (w335:u32[])
                      n66 = local read "All ID list 2"() -> (w330:u32[])
                      n67 = local read "All ID list 1"() -> (w337:u32[])
                      n68 = case shown="True" w331 {
                        tunnel: [w364 w378] -> w326
                        tunnel: w341 -> [_ w377]
                        tunnel: w340 -> [w364 w376]
                        tunnel: [w363 w373] -> w339
                        tunnel: w320 -> [_ w372]
                        tunnel: w319 -> [_ w371]
                        tunnel: w318 -> [_ w370]
                        tunnel: [_ w369] -> w317
                        tunnel: w337 -> [_ w366]
                        tunnel: w336 -> [_ w367]
                        tunnel: w335 -> [_ w368]
                        tunnel: w332 -> [w363 _]
                        tunnel: w312 -> [_ w365]
                        frame False {
                          # "Hardware 1 not enabled"
                        }
                        frame True {
                          # "Hardware 1 enabled"
                          n69 = call "PixelReg ProgramFromFile 2nPas.vi"("connection ID"=w377, "ACQ PxReg folder"=w370, "EQ folder path"=w371, "PixelReg (hex)"=w372, "All ID list"=w366, "Layer ID list"=w367, "Chip ID list"=w368, "error in (no error)"=w376, "PA gain"=w365) -> ("connection ID out"=w375:refnum<k5>, "done message"=w369:string, "All checks OK"=w373:bool, "error out (no error)"=w374:errorcluster)  [unwired: 2 in, 1 out]
                          n70 = call "CloseEthConnection.vi"("error in (no error)"=w374, "connection ID"=w375) -> ("error out"=w378:errorcluster)  [unwired: 9 in]
                        }
                      }
                      n71 = case shown="True" w332 {
                        tunnel: [w348 w362] -> w325
                        tunnel: w334 -> [_ w361]
                        tunnel: w333 -> [w348 w360]
                        tunnel: [w347 w357] -> w323
                        tunnel: w320 -> [_ w356]
                        tunnel: w319 -> [_ w355]
                        tunnel: w318 -> [_ w354]
                        tunnel: [_ w353] -> w313
                        tunnel: w330 -> [_ w350]
                        tunnel: w329 -> [_ w351]
                        tunnel: w328 -> [_ w352]
                        tunnel: w331 -> [w347 _]
                        tunnel: w312 -> [_ w349]
                        frame False {
                          # "Hardware 2 not enabled"
                        }
                        frame True {
                          # "Hardware 2 enabled"
                          n72 = call "PixelReg ProgramFromFile 2nPas.vi"("connection ID"=w361, "ACQ PxReg folder"=w354, "EQ folder path"=w355, "PixelReg (hex)"=w356, "All ID list"=w350, "Layer ID list"=w351, "Chip ID list"=w352, "error in (no error)"=w360, "PA gain"=w349) -> ("connection ID out"=w359:refnum<k5>, "done message"=w353:string, "All checks OK"=w357:bool, "error out (no error)"=w358:errorcluster)  [unwired: 2 in, 1 out]
                          n73 = call "CloseEthConnection.vi"("error in (no error)"=w358, "connection ID"=w359) -> ("error out"=w362:errorcluster)  [unwired: 9 in]
                        }
                      }
                      n74 = Merge Errors(w326, w325) -> (w327:errorcluster)
                      n75 = call <vilib>:"Simple Error Handler.vi"("error in (no error)"=w327) -> ()  [unwired: 4 in, 5 out]
                      n76 = Unbundle By Name(w327) -> ("status"=w342:bool)
                      n77 = Concatenate Strings "Concatenate Strings"(w322, w321, w317, w316, w316, w315, w314, w313) -> (w345:string)
                      n78 = Compound Arithmetic op=AND(invert w342, w339, w324, w323) -> (w344:bool)
                      n79 = property on="Error tick" class="Bool (strict)"(reference=w343, "Value"=w342) -> ()  [unwired: 1 in, 2 out]
                      n80 = case shown="True" w344 {
                        tunnel: w345 -> [_ w388]
                        frame False {
                          # "error"
                        }
                        frame True {
                          # "OK x3"
                          n81 = call "MessageTimeOk.vi"("time (ms)"=5200, "missage"=w388) -> ()  [unwired: 4 in]
                        }
                      }
                    }
                  }
                }
              }
            }
            frame #1 {
              w396 = u32 0 ("Value")
              # "Mostra quina EQualització carrega"
              # "Llegeix HV final value from EQ loaded"
              # "Inicialitza variables 'actual time'"
              # "1) Inicialitzacions a la Adquisició. Ask for comments"
              n82 = flat-sequence {
                tunnel: w411 -> [w426]
                tunnel: [w425] -> w407
                tunnel: [w424] -> w405
                tunnel: w404 -> [w424]
                tunnel: [w430] -> w409
                tunnel: [w429] -> w408
                tunnel: w407 -> [w429]
                tunnel: w405 -> [w428]
                tunnel: [w433] -> w406
                tunnel: w409 -> [w433]
                tunnel: w408 -> [w432]
                frame #0 {
                  n83 = property on="Operation text" class="Str"(reference=w426, "Value"="Acquiring...\nWrite comments for file.") -> (reference out=w425:refnum<vi>)  [unwired: 1 in, 1 out]
                }
                frame #1 {
                  # "ask for comments"
                  n84 = call "Acq_askComents.vi"("Folder path"=w428) -> ("Complete file path"=w430:path)  [unwired: 4 in]
                }
                frame #2 {
                  n85 = property on="Operation text" class="Str"(reference=w432, "Value"="Acquiring...") -> ()  [unwired: 1 in, 2 out]
                }
              }
              n86 = property on="etapa2 Actual time" class="DigNum (strict)"(reference=w421, "Value"=w396) -> ()  [unwired: 1 in, 2 out]
              n87 = property on="etapa5 Actual time" class="DigNum (strict)"(reference=w419, "Value"=w396) -> ()  [unwired: 1 in, 2 out]
              n88 = property on="Events fets" class="DigNum (strict)"(reference=w399, "Value"=w396) -> ()  [unwired: 1 in, 2 out]
              n89 = property on="Events fets A" class="DigNum (strict)"(reference=w398, "Value"=w396) -> ()  [unwired: 1 in, 2 out]
              n90 = property on="Events fets B" class="DigNum (strict)"(reference=w397, "Value"=w396) -> ()  [unwired: 1 in, 2 out]
              n91 = property on="etapa3 Actual time" class="DigNum (strict)"(reference=w420, "Value"=w396) -> ()  [unwired: 1 in, 2 out]
              n92 = property on="HV parameters" class="Clust (strict)"(reference=w418) -> (reference out=w415:refnum<vi>, "Value"=w417:T5)  [unwired: 1 in, 1 out]
              n93 = property on="Stop ACQ button" class="Bool (strict)"(reference=w403, "Value"=FALSE, "DisabledEnum"=T4."Enabled" ("Disabled"), "Visible"=TRUE) -> ()  [unwired: 1 in, 2 out]
              n94 = in-place {
                in-place-border: w410 -> [w434]
                n95 = in-place-cluster #1(w417) -> ()  [unwired: 1 out]
                n96 = in-place-cluster #1("Final value"=w434) -> (w416:T5)
              }
              n97 = String To Path(string=w412) -> (path=w413:path)
              n98 = property class="Path"(reference="EQ folder path Refnum", "Value"=w413) -> ()  [unwired: 1 in, 2 out]
              n99 = property on="HV parameters" class="Clust (strict)"(reference=w415, "Value"=w416) -> ()  [unwired: 1 in, 2 out]
              n100 = property on="Motors" class="Clust (strict)"(reference=w395) -> (reference out=w393:refnum<vi>, error out=w392:errorcluster, "Value"=w391:T6)  [unwired: 1 in]
              n101 = Unbundle By Name(w391) -> ("Vertical motor"=w394:bool)
              n102 = case "Get initial vertical position" shown="True" w394 {
                tunnel: [_ w422] -> w390
                frame False {
                }
                frame True {
                  w423 = u8 14 items=["rotating"=6, "vertical"=14] ("motor")
                  n103 = call "dr_M_GetPOS_rotate&vertical.vi"("motor"=w423) -> ("POSition"=w422:u32)  [unwired: 9 in, 1 out]
                }
              }
              n104 = Bundle By Name(cluster=w391, "vertical position"=w390) -> (w389:T6)
              n105 = property on="Motors" class="Clust (strict)"(reference=w393, error in=w392, "Value"=w389) -> ()  [unwired: 2 out]
            }
            frame #2 {
              w436 = u32 0  # Comptador events per file
              w444 = u32 1  # first file sufix num.
              # "Desactiva busy per permetre\nmesura de temperatura\ndurant ACQ data viewer."
              # "2) ADQUISICIÓ"
              n106 = while {
                tunnel: w465 -> [w497]
                tunnel: w464 -> [w496]
                tunnel: w463 -> [w495]
                tunnel: w462 -> [w494]
                tunnel: w461 -> [w493]
                tunnel: w460 -> [w492]
                tunnel: w459 -> [w491]
                tunnel: w458 -> [w490]
                tunnel: w457 -> [w489]
                tunnel: w456 -> [w488]
                tunnel: w455 -> [w487]
                tunnel: w454 -> [w486]
                tunnel: w453 -> [w485]
                tunnel: w443 -> [w484]
                tunnel: w452 -> [w483]
                tunnel: w451 -> [w482]
                tunnel: [w481] -> w450
                tunnel: w449 -> [w479]
                tunnel: w448 -> [w478]
                tunnel: w447 -> [w477]
                tunnel: [w476] -> w445
                shift-right: [w474] -> _
                shift-left: w444 -> [w475]
                tunnel: [w473] -> w442
                shift-right: [w471] -> w439
                shift-left: u32 0 -> [w472]
                tunnel: w438 -> [w470]
                tunnel: w437 -> [w469]
                shift-right: [w467] -> _
                shift-left: w436 -> [w468]
                tunnel: w435 -> [w466]
                i -> [w473]
                stop <- w480 stop-if-true
                n107 = stacked-sequence {
                  tunnel: w497 -> [_ _ w555 _ _ _ _ _ _ _]
                  tunnel: w496 -> [_ _ w557 _ _ _ _ _ _ _]
                  tunnel: w495 -> [w501 _ w556 _ _ _ _ _ _ _]
                  tunnel: w494 -> [_ _ _ _ w632 _ _ _ _ w860]
                  tunnel: w493 -> [w500 _ _ _ w631 _ _ _ _ _]
                  tunnel: w492 -> [_ _ _ _ _ _ _ _ w806 _]
                  tunnel: w491 -> [_ _ _ _ _ _ _ _ w807 _]
                  tunnel: w490 -> [w499 _ _ _ _ _ _ _ w805 _]
                  tunnel: w489 -> [_ w513 _ _ _ _ w723 _ _ _]
                  tunnel: w488 -> [_ w506 _ _ _ _ w722 _ _ _]
                  tunnel: w487 -> [_ w509 _ _ w634 _ w721 _ _ _]
                  tunnel: w486 -> [_ w504 _ _ _ _ w720 _ _ _]
                  tunnel: w485 -> [_ w514 w554 w600 w630 w682 w714 w756 w804 w863]
                  tunnel: w484 -> [_ w511 w553 _ _ _ w717 _ w803 _]
                  tunnel: w483 -> [_ _ _ _ w636 _ _ _ _ _]
                  tunnel: w482 -> [_ _ _ _ w635 _ _ _ w798 _]
                  tunnel: [_ _ _ _ w633 _ _ _ _ _] -> w481
                  tunnel: [_ _ _ _ _ _ _ _ _ w862] -> w480
                  tunnel: w479 -> [_ _ _ _ w628 _ _ _ _ _]
                  tunnel: w478 -> [_ w503 w551 _ w624 _ w715 _ w801 w861]
                  tunnel: w477 -> [_ _ w549 _ _ _ _ _ w799 _]
                  tunnel: [_ _ _ _ _ _ _ _ _ w861] -> w476
                  tunnel: w475 -> [_ _ _ _ _ _ _ _ w790 _]
                  tunnel: [_ _ _ _ _ _ _ _ w797 _] -> w474
                  tunnel: w472 -> [_ _ _ _ _ _ _ _ _ w859]
                  tunnel: [_ _ _ _ _ _ _ _ _ w857] -> w471
                  tunnel: w470 -> [_ _ _ _ w627 _ _ _ _ _]
                  tunnel: w469 -> [_ _ _ _ w626 _ _ _ _ _]
                  tunnel: w468 -> [_ _ _ _ _ _ _ _ w791 _]
                  tunnel: [_ _ _ _ _ _ _ _ w796 _] -> w467
                  tunnel: w466 -> [_ _ _ w599 _ w683 _ w757 _ _]
                  frame #0 {
                    w498 = u8 0 ("ACQ-e2 barra")
                    # "Inicialitzacions a la iteració"
                    n108 = property on="etapa2 barra" class="Slide (strict)"(reference=w501, "Value"=w498) -> ()  [unwired: 1 in, 2 out]
                    n109 = property on="etapa3 barra" class="Slide (strict)"(reference=w500, "Value"=w498) -> ()  [unwired: 1 in, 2 out]
                    n110 = property on="etapa5 barra" class="Slide (strict)"(reference=w499, "Value"=w498) -> ()  [unwired: 1 in, 2 out]
                  }
                  frame #1 {
                    # "Etapa 1:  rampa pujada HV"
                    n111 = flat-sequence {
                      tunnel: w514 -> [w515]
                      tunnel: w513 -> [w520]
                      tunnel: [w523] -> w512
                      tunnel: w511 -> [w522]
                      tunnel: [w521] -> w510
                      tunnel: w509 -> [w521]
                      tunnel: [w520] -> w508
                      tunnel: [w519] -> w507
                      tunnel: w506 -> [w519]
                      tunnel: [w518] -> w505
                      tunnel: w504 -> [w518]
                      tunnel: w503 -> [w516]
                      tunnel: [w515] -> w502
                      frame #0 {
                        # "Desactiva busy per permetre\nmesura de temperatura\ndurant rampa HV i temps H"
                        n112 = property on="HV level" class="Slide (strict)"(reference=w520) -> ("Value"=w526:dbl)  [unwired: 1 in, 2 out]
                        n113 = property on="Stop ACQ" class="Bool (strict)"(reference=w515) -> ("Value"=w524:bool)  [unwired: 1 in, 2 out]
                        n114 = property on="busy = F" class="Bool (strict)"(reference=w516, "Value"=FALSE) -> ()  [unwired: 1 in, 2 out]
                        n115 = Not Equal To 0?(x=w526) -> (x != 0?=w525:bool)
                        n116 = Compound Arithmetic op=OR "OR"(w525, w524, invert w522) -> (w523:bool)
                      }
                    }
                    n117 = case shown="False" w512 {
                      tunnel: w507 -> [w534 _]
                      tunnel: w508 -> [w531 _]
                      tunnel: w510 -> [w530 _]
                      tunnel: w505 -> [w528 _]
                      tunnel: w502 -> [w527 _]
                      frame False {
                        n118 = flat-sequence {
                          tunnel: [w543] -> w537
                          tunnel: w534 -> [w548]
                          tunnel: [w546] -> w533
                          tunnel: [w545] -> w532
                          tunnel: w528 -> [w542]
                          frame #0 {
                            n119 = property on="HV parameters" class="Clust (strict)"(reference=w542) -> ("Value"=w543:T5)  [unwired: 1 in, 2 out]
                            n120 = property on="HV string" class="Str"(reference=w548, "Value"="HV ramping" ("HV String"), "Text.FontColor"=u32 15365376) -> (reference out=w546:refnum<vi>, error out=w545:errorcluster)  [unwired: 1 in]
                          }
                        }
                        n121 = call "HV_drive.vi"("Stop subVI Refnum"=w527, "HV level Refnum"=w531, "HV parameters"=w537) -> ("error out"=w536:errorcluster, "HV level (last value)"=w535:dbl)  [unwired: 1 in]
                        n122 = flat-sequence {
                          tunnel: w535 -> [_]
                          tunnel: w533 -> [w540]
                          tunnel: w532 -> [w539]
                          frame #0 {
                            n123 = property on="HV string" class="Str"(reference=w540, error in=w539, "Value"="HV presence!" ("HV String"), "Text.FontColor"=u32 16711680) -> ()  [unwired: 2 out]
                          }
                        }
                        n124 = Unbundle By Name(w536) -> ("status"=w529:bool)
                        n125 = call <vilib>:"Simple Error Handler.vi"("error in (no error)"=w536) -> ()  [unwired: 4 in, 5 out]
                        n126 = property on="Error tick" class="Bool (strict)"(reference=w530, "Value"=w529) -> ()  [unwired: 1 in, 2 out]
                      }
                      frame True {
                        # "executant aturada\no hi ha HV manual\no HV not enabled"
                      }
                    }
                  }
                  frame #2 {
                    # "Etapa 2:  temps inicial a HV_H"
                    n127 = flat-sequence {
                      tunnel: w557 -> [w564]
                      tunnel: w556 -> [w563]
                      tunnel: w555 -> [w562]
                      tunnel: w554 -> [w561]
                      tunnel: w553 -> [w560]
                      tunnel: [w559] -> w552
                      tunnel: w551 -> [w559]
                      tunnel: [w558] -> w550
                      tunnel: w549 -> [w558]
                      tunnel: w552 -> [w593]
                      tunnel: w550 -> [w592]
                      frame #0 {
                        n128 = case shown="True" w560 {
                          tunnel: w564 -> [_ w570]
                          tunnel: w563 -> [_ w568]
                          tunnel: w562 -> [_ w567]
                          tunnel: w561 -> [_ w566]
                          frame False {
                          }
                          frame True {
                            n129 = property on="etapa2 Actual time" class="DigNum (strict)"(reference=w570, "Value"=u32 0 ("ACQ-e2 Actual time")) -> (reference out=w569:refnum<vi>)  [unwired: 1 in, 1 out]
                            n130 = Tick Count (ms)() -> (millisecond timer value=w571:u32)
                            n131 = while {
                              tunnel: w571 -> [w590]
                              tunnel: w569 -> [w580]
                              tunnel: w567 -> [w579]
                              tunnel: w568 -> [w577]
                              tunnel: w566 -> [w573]
                              stop <- w575 stop-if-true
                              n132 = property on="etapa2 Waiting time" class="DigNum (strict)"(reference=w579) -> ("Value"=w578:u32)  [unwired: 1 in, 2 out]
                              n133 = Tick Count (ms)() -> (millisecond timer value=w591:u32)
                              n134 = property on="Stop ACQ" class="Bool (strict)"(reference=w573) -> ("Value"=w572:bool)  [unwired: 1 in, 2 out]
                              n135 = Subtract(x=w591, y=w590) -> (x-y=w589:u32)
                              n136 = Quotient & Remainder(x=w589, y=u32 1000) -> (floor(x/y)=w581:u32)  [unwired: 1 out]
                              n137 = Greater Or Equal?(x=w581, y=w578) -> (x >= y?=w574:bool)
                              n138 = To Double Precision Float(number=w581) -> (double precision float=w582:dbl)
                              n139 = To Double Precision Float(number=w578) -> (double precision float=w583:dbl)
                              n140 = property on="etapa2 Actual time" class="DigNum (strict)"(reference=w580, "Value"=w581) -> ()  [unwired: 1 in, 2 out]
                              n141 = Divide(x=w582, y=w583) -> (x/y=w586:dbl)
                              n142 = Or(x=w574, y=w572) -> (x .or. y?=w575:bool)
                              n143 = Multiply(x=w586, y=100.0) -> (x*y=w584:dbl)
                              n144 = To Unsigned Byte Integer(number=w584) -> (unsigned 8bit integer=w576:u8)
                              n145 = property on="etapa2 barra" class="Slide (strict)"(reference=w577, "Value"=w576) -> ()  [unwired: 1 in, 2 out]
                              n146 = Wait Until Next ms Multiple(millisecond multiple=u32 100) -> ()  [unwired: 1 out]
                            }
                          }
                        }
                      }
                      frame #1 {
                        # "Reactiva busy per procedir a l'adquisició"
                        n147 = flat-sequence {
                          tunnel: w593 -> [w597]
                          tunnel: w592 -> [w595]
                          tunnel: [w595] -> w594
                          tunnel: w594 -> [w598]
                          frame #0 {
                            n148 = property on="busy = T" class="Bool (strict)"(reference=w597, "Value"=TRUE) -> ()  [unwired: 1 in, 2 out]
                          }
                          frame #1 {
                            n149 = Wait (ms)(milliseconds to wait=w598) -> ()  [unwired: 1 out]
                          }
                        }
                      }
                    }
                  }
                  frame #3 {
                    # "Motors ON"
                    n150 = disable-structure shown="Disabled" {
                      disable-tunnel: w600 -> [w611 _]
                      disable-tunnel: w599 -> [w610 _]
                      frame Disabled {
                        n151 = property on="Stop ACQ button" class="Bool (strict)"(reference=w611) -> (reference out=w602:refnum<vi>, "Value"=w603:bool)  [unwired: 1 in, 1 out]
                        n152 = property on="Motors" class="Clust (strict)"(reference=w610) -> ("Value"=w609:T6)  [unwired: 1 in, 2 out]
                        n153 = Unbundle By Name(w609) -> ("Rotation motor"=w605:bool, "Vertical motor"=w608:bool)
                        n154 = Compound Arithmetic op=AND "AND"(w608, invert w603) -> (w607:bool)
                        n155 = case shown="True" w607 {
                          tunnel: [_ w620] -> w604
                          frame False {
                          }
                          frame True {
                            w621 = "20"  # SPEED (12k)
                            w622 = 1000000  # Position
                            # "Start vertical motor"
                            n156 = call "dr_M_vertical.vi"("SPEED (12k)"=w621, "Position"=w622) -> ("error out"=w620:errorcluster)  [unwired: 9 in]
                          }
                        }
                        n157 = Compound Arithmetic op=AND "AND"(w605, invert w603) -> (w606:bool)
                        n158 = case shown="True" w606 {
                          tunnel: w604 -> [w615 w619]
                          tunnel: [w615 w618] -> w601
                          frame False {
                          }
                          frame True {
                            w616 = "1"  # SPEED (500)
                            w617 = 40000  # Step
                            # "Start rotation motor"
                            n159 = call "dr_M_rotate.vi"("error in"=w619, "SPEED (500)"=w616, "movement"=w617) -> ("error out"=w618:errorcluster)  [unwired: 8 in]
                          }
                        }
                        n160 = case shown="Error" w601 {
                          selector: w601 -> [_ w613]
                          tunnel: w602 -> [_ w614]
                          frame No Error {
                          }
                          frame Error {
                            n161 = Unbundle By Name(w613) -> ("status"=w612:bool)
                            n162 = property on="Stop ACQ button" class="Bool (strict)"(reference=w614, "Value"=w612) -> ()  [unwired: 1 in, 2 out]
                          }
                        }
                      }
                      frame Enabled {
                      }
                    }
                  }
                  frame #4 {
                    # "Etapa 3:  adquisició"
                    n163 = property on="Stop ACQ button" class="Bool (strict)"(reference=w630) -> ("Value"=w629:bool)  [unwired: 1 in, 2 out]
                    n164 = property on="busy = T" class="Bool (strict)"(reference=w624, "Value"=TRUE) -> (reference out=w623:refnum<vi>)  [unwired: 1 in, 1 out]
                    n165 = case shown="False" w629 {
                      tunnel: w636 -> [w647 _]
                      tunnel: w635 -> [w639 _]
                      tunnel: w634 -> [w656 _]
                      tunnel: w630 -> [w652 _]
                      tunnel: [w642 _] -> w633
                      tunnel: w632 -> [w648 _]
                      tunnel: w631 -> [w649 _]
                      tunnel: w628 -> [w646 _]
                      tunnel: w627 -> [w638 _]
                      tunnel: w626 -> [w637 _]
                      tunnel: w623 -> [_ _]
                      frame False {
                        # "si no hi ha Stop ordenat, adquireix"
                        n166 = in-place "Conversion of DTP: ms to comptes" {
                          n167 = in-place-cluster #2("ACQ Parameters (cluster)") -> ("DTP period"=w676:u32)
                          n168 = To Double Precision Float(number=w676) -> (double precision float=w677:dbl)
                          n169 = Divide(x=w677, y=2.5e-05) -> (x/y=w680:dbl)
                          n170 = Decrement(x=w680) -> (x-1=w679:dbl)
                          n171 = To Unsigned Long Integer(number=w679) -> (unsigned 32bit integer=w678:u32)
                          n172 = in-place-cluster #2("DTP period"=w678) -> (w662:T2)
                        }
                        n173 = property class="DigNum (strict)"(reference="Events to acquire Refnum") -> ("Value"=w658:u32)  [unwired: 1 in, 2 out]
                        n174 = local read "Addresses Cluster"() -> (w640:T1)
                        n175 = Cluster To Array(cluster=w662) -> (array=w650:u32[])
                        n176 = Bundle(TRUE, "Value"=w658) -> (w651:cluster{bool, "Value":u32})  [unwired: 1 in]
                        n177 = call "subop_x2_Acquisition.vi"("ACQ stop by events"=w651, "ACQ parameters"=w650, "events fets A Refnum"=w638, "events fets B Refnum"=w637, "Base file path"=w639, "Addresses Cluster"=w640, "Stop ACQ button Refnum"=w652, "ACQ barra Refnum"=w649, "Actual time Refnum"=w648, "Acquisition time Refnum"=w647, "Total events Refnum"=w646) -> ("Stop by events"=w641:bool, "ACQ WatchDog timeout"=w642:bool, "ACQ Answer 1i2"=w643:string, "error out comm"=w645:errorcluster, "error out file"=w644:errorcluster)  [unwired: 12 in]
                        n178 = Or(x=w642, y=w641) -> (x .or. y?=w653:bool)
                        n179 = flat-sequence {
                          tunnel: w653 -> [w664]
                          tunnel: w652 -> [w663]
                          tunnel: w642 -> [w668]
                          frame #0 {
                            n180 = case shown="True" w664 {
                              tunnel: w663 -> [_ w667]
                              frame False {
                              }
                              frame True {
                                # "Stop by events   /or/\nWatchdog: stop execution"
                                n181 = property on="Stop ACQ button" class="Bool (strict)"(reference=w667, "Value"=TRUE, "DisabledEnum"=T4."Disabled" ("Disabled")) -> ()  [unwired: 1 in, 2 out]
                              }
                            }
                          }
                          frame #1 {
                            n182 = case shown="True" w668 {
                              frame False {
                              }
                              frame True {
                                n183 = call "MessageTimeOk.vi"("time (ms)"=10000, "missage"="Acquisition WatchDog timeout." ("message")) -> ()  [unwired: 4 in]
                              }
                            }
                          }
                        }
                        n184 = Merge Errors(w645, w644) -> (w657:errorcluster)
                        n185 = call <vilib>:"Simple Error Handler.vi"("error in (no error)"=w657) -> ()  [unwired: 4 in, 5 out]
                        n186 = Unbundle By Name(w657) -> ("status"=w655:bool)
                        n187 = property on="Error tick" class="Bool (strict)"(reference=w656, "Value"=w655) -> ()  [unwired: 1 in, 2 out]
                        n188 = Or(x=w644, y=w642) -> (x .or. y?=w654:bool)
                        n189 = case shown="False" w654 {
                          tunnel: w643 -> [w671 _]
                          frame False {
                            # "No hi ha errors file"
                            n190 = Concatenate Strings(w671, "\r", "The files have been saved.") -> (w674:string)
                            n191 = call "MessageTimeOk.vi"("time (ms)"=3500, "missage"=w674) -> ()  [unwired: 4 in]
                          }
                          frame True {
                            # "Algun error"
                          }
                        }
                      }
                      frame True {
                        # "Stop ordenat"
                      }
                    }
                  }
                  frame #5 {
                    # "Motors OFF"
                    n192 = disable-structure shown="Disabled" {
                      disable-tunnel: w683 -> [w691 _]
                      disable-tunnel: w682 -> [w685 _]
                      frame Disabled {
                        n193 = property on="Motors" class="Clust (strict)"(reference=w691) -> (reference out=w684:refnum<vi>, "Value"=w687:T6)  [unwired: 1 in, 1 out]
                        n194 = Unbundle By Name(w687) -> ("Vertical motor"=w688:bool, "Rotation motor"=w690:bool)
                        n195 = Or(x=w688, y=w690) -> (x .or. y?=w689:bool)
                        n196 = case shown="True" w689 {
                          tunnel: [_ w713] -> w686
                          frame False {
                          }
                          frame True {
                            n197 = call "dr_M_STOP_rotate&vertical.vi"() -> ("error out"=w713:errorcluster)  [unwired: 11 in]
                          }
                        }
                        n198 = case shown="No Error" w686 {
                          selector: w686 -> [w694 _]
                          tunnel: w688 -> [w696 _]
                          tunnel: w687 -> [w695 _]
                          tunnel: w685 -> [w693 w712]
                          tunnel: w684 -> [w692 _]
                          frame No Error {
                            n199 = case shown="True" w696 {
                              tunnel: w695 -> [_ w699]
                              tunnel: w694 -> [_ w708]
                              tunnel: w693 -> [_ w704]
                              tunnel: w692 -> [_ w700]
                              frame False {
                              }
                              frame True {
                                w707 = u8 14 items=["rotating"=6, "vertical"=14] ("motor")
                                # "Stop ACQ?"
                                n200 = Unbundle By Name(w699) -> ("Final vertical position"=w701:u32)
                                n201 = call "dr_M_GetPOS_rotate&vertical.vi"("error in"=w708, "motor"=w707) -> ("error out"=w706:errorcluster, "POSition"=w698:u32)  [unwired: 8 in]
                                n202 = Bundle By Name(cluster=w699, "vertical position"=w698) -> (w697:T6)
                                n203 = Unbundle By Name(w706) -> ("status"=w705:bool)
                                n204 = Greater Or Equal?(x=w698, y=w701) -> (x >= y?=w703:bool)
                                n205 = Or(x=w703, y=w705) -> (x .or. y?=w702:bool)
                                n206 = property class="Clust (strict)"(reference=w700, "Value"=w697) -> ()  [unwired: 1 in, 2 out]
                                n207 = case shown="True" w702 {
                                selector: w702 -> [_ w709]
                                tunnel: w704 -> [_ w710]
                                frame False {
                                }
                                frame True {
                                n208 = property on="Stop ACQ button" class="Bool (strict)"(reference=w710, "Value"=w709) -> ()  [unwired: 1 in, 2 out]
                                }
                                }
                              }
                            }
                          }
                          frame Error {
                            n209 = property on="Stop ACQ button" class="Bool (strict)"(reference=w712, "Value"=TRUE) -> ()  [unwired: 1 in, 2 out]
                          }
                        }
                      }
                      frame Enabled {
                      }
                    }
                  }
                  frame #6 {
                    # "Tant si hi ha Stop adquisició ordenat com si no, executa rampa baixada HV"
                    # "Etapa 4:  rampa bajada HV"
                    n210 = flat-sequence {
                      tunnel: w717 -> [w727]
                      tunnel: [w727] -> w716
                      tunnel: w715 -> [w725]
                      frame #0 {
                        # "Desactiva busy per permetre\nmesura de temperatura\ndurant rampa HV i temps L"
                        n211 = property on="busy = F" class="Bool (strict)"(reference=w725, "Value"=FALSE) -> ()  [unwired: 1 in, 2 out]
                      }
                    }
                    n212 = property on="HV level" class="Slide (strict)"(reference=w723) -> ("Value"=w724:dbl)  [unwired: 1 in, 2 out]
                    n213 = Not Equal To 0?(x=w724) -> (x != 0?=w719:bool)
                    n214 = And(x=w719, y=w716) -> (x .and. y?=w718:bool)
                    n215 = case shown="True" w718 {
                      tunnel: w723 -> [_ w732]
                      tunnel: w722 -> [_ w731]
                      tunnel: w721 -> [_ w730]
                      tunnel: w720 -> [_ w729]
                      tunnel: w714 -> [_ w728]
                      frame False {
                        # "HV = 0,   no cal baixada"
                      }
                      frame True {
                        n216 = flat-sequence {
                          tunnel: [w749] -> w733
                          tunnel: w731 -> [w755]
                          tunnel: [w753] -> w736
                          tunnel: [w752] -> w737
                          tunnel: w729 -> [w750]
                          frame #0 {
                            n217 = property on="HV parameters" class="Clust (strict)"(reference=w750) -> ("Value"=w749:T5)  [unwired: 1 in, 2 out]
                            n218 = property on="HV string" class="Str"(reference=w755, "Value"="HV ramping" ("HV String"), "Text.FontColor"=u32 15365376) -> (reference out=w753:refnum<vi>, error out=w752:errorcluster)  [unwired: 1 in]
                          }
                        }
                        n219 = call "HV_drive.vi"("Stop subVI Refnum"=w728, "HV level Refnum"=w732, "HV parameters"=w733) -> ("error out"=w734:errorcluster, "HV level (last value)"=w735:dbl)  [unwired: 1 in]
                        n220 = flat-sequence {
                          tunnel: w735 -> [w741]
                          tunnel: w736 -> [w748]
                          tunnel: w737 -> [w747]
                          frame #0 {
                            n221 = Equal To 0?(x=w741) -> (x = 0?=w746:bool)
                            n222 = Select(t="HV off", s=w746, f="HV presence!") -> (s? t:f=w740:string)
                            n223 = Select(t=u32 42533, s=w746, f=u32 16711680) -> (s? t:f=w739:u32)
                            n224 = property on="HV string" class="Str"(reference=w748, error in=w747, "Value"=w740, "Text.FontColor"=w739) -> ()  [unwired: 2 out]
                          }
                        }
                        n225 = Unbundle By Name(w734) -> ("status"=w738:bool)
                        n226 = call <vilib>:"Simple Error Handler.vi"("error in (no error)"=w734) -> ()  [unwired: 4 in, 5 out]
                        n227 = property on="Error tick" class="Bool (strict)"(reference=w730, "Value"=w738) -> ()  [unwired: 1 in, 2 out]
                      }
                    }
                  }
                  frame #7 {
                    # "Motors: move a step"
                    n228 = disable-structure shown="Disabled" {
                      disable-tunnel: w757 -> [w760 _]
                      disable-tunnel: w756 -> [w759 _]
                      frame Disabled {
                        n229 = property on="Motors" class="Clust (strict)"(reference=w760) -> (reference out=w761:refnum<vi>, "Value"=w762:T6)  [unwired: 1 in, 1 out]
                        n230 = Unbundle By Name(w762) -> ("Vertical motor"=w763:bool, "Rotation motor"=w764:bool)
                        n231 = And(x=w763, y=w764) -> (x .and. y?=w758:bool)
                        n232 = case shown="True" w758 {
                          tunnel: w762 -> [_ w775]
                          tunnel: w759 -> [_ w786]
                          tunnel: w761 -> [_ w773]
                          frame False {
                          }
                          frame True {
                            w785 = u8 14 items=["rotating"=6, "vertical"=14] ("motor")
                            n233 = Unbundle By Name(w775) -> ("Final vertical position"=w784:u32)
                            n234 = call "dr_M_GetPOS_rotate&vertical.vi"("motor"=w785) -> ("error out"=w778:errorcluster, "POSition"=w774:u32)  [unwired: 9 in]
                            n235 = Greater Or Equal?(x=w774, y=w784) -> (x >= y?=w768:bool)
                            n236 = Bundle By Name(cluster=w775, "vertical position"=w774) -> (w772:T6)
                            n237 = Add(x=w774, y=u32 1311) -> (x+y=w783:u32)
                            n238 = Select(t=u32 297215, s=w768, f=w783) -> (s? t:f=w781:u32)
                            n239 = To Long Integer(number=w781) -> (32bit integer=w780:i32)
                            n240 = property class="Clust (strict)"(reference=w773, "Value"=w772) -> ()  [unwired: 1 in, 2 out]
                            n241 = call "dr_M_vertical.vi"("error in"=w778, "SPEED (12k)"="1200", "Position"=w780) -> ("error out"=w770:errorcluster)  [unwired: 8 in]
                            n242 = Select(t=100000, s=w768, f=64 ("movement")) -> (s? t:f=w766:i32)
                            n243 = call "dr_M_rotate.vi"("error in"=w770, "SPEED (500)"="200", "movement"=w766, "type of mov. (F)"=w768) -> ("error out"=w769:errorcluster)  [unwired: 7 in]
                            n244 = Unbundle By Name(w769) -> ("status"=w777:bool)
                            n245 = case shown="True" w777 {
                              selector: w777 -> [_ w787]
                              tunnel: w786 -> [_ w788]
                              frame False {
                              }
                              frame True {
                                n246 = property on="Stop ACQ button" class="Bool (strict)"(reference=w788, "Value"=w787) -> ()  [unwired: 1 in, 2 out]
                              }
                            }
                          }
                        }
                      }
                      frame Enabled {
                      }
                    }
                  }
                  frame #8 {
                    # "Etapa 5:  temps final a HV_L"
                    n247 = local read "Chip ID list 1"() -> (w794:u32[])
                    n248 = local read "Chip ID list 2"() -> (w795:u32[])
                    n249 = flat-sequence {
                      tunnel: w807 -> [w822]
                      tunnel: w806 -> [w821]
                      tunnel: w805 -> [w820]
                      tunnel: w804 -> [w819]
                      tunnel: w803 -> [w818]
                      tunnel: [w817] -> w802
                      tunnel: w801 -> [w817]
                      tunnel: [w816] -> w800
                      tunnel: w799 -> [w816]
                      tunnel: w802 -> [w851]
                      tunnel: w800 -> [w850]
                      frame #0 {
                        n250 = case shown="True" w818 {
                          tunnel: w822 -> [_ w829]
                          tunnel: w821 -> [_ w826]
                          tunnel: w820 -> [_ w825]
                          tunnel: w819 -> [_ w824]
                          frame False {
                          }
                          frame True {
                            n251 = property on="etapa5 Actual time" class="DigNum (strict)"(reference=w829, "Value"=u32 0 ("ACQ-e2 Actual time")) -> (reference out=w827:refnum<vi>)  [unwired: 1 in, 1 out]
                            n252 = Tick Count (ms)() -> (millisecond timer value=w828:u32)
                            n253 = while {
                              tunnel: w828 -> [w848]
                              tunnel: w827 -> [w838]
                              tunnel: w826 -> [w837]
                              tunnel: w825 -> [w835]
                              tunnel: w824 -> [w831]
                              stop <- w833 stop-if-true
                              # "et5: temps final a HV_L"
                              n254 = property on="etapa5 Waiting time" class="DigNum (strict)"(reference=w837) -> ("Value"=w836:u32)  [unwired: 1 in, 2 out]
                              n255 = Tick Count (ms)() -> (millisecond timer value=w849:u32)
                              n256 = property on="Stop ACQ" class="Bool (strict)"(reference=w831) -> ("Value"=w830:bool)  [unwired: 1 in, 2 out]
                              n257 = Subtract(x=w849, y=w848) -> (x-y=w847:u32)
                              n258 = Quotient & Remainder(x=w847, y=u32 1000) -> (floor(x/y)=w839:u32)  [unwired: 1 out]
                              n259 = Greater Or Equal?(x=w839, y=w836) -> (x >= y?=w832:bool)
                              n260 = To Double Precision Float(number=w839) -> (double precision float=w840:dbl)
                              n261 = To Double Precision Float(number=w836) -> (double precision float=w841:dbl)
                              n262 = property on="etapa5 Actual time" class="DigNum (strict)"(reference=w838, "Value"=w839) -> ()  [unwired: 1 in, 2 out]
                              n263 = Or(x=w832, y=w830) -> (x .or. y?=w833:bool)
                              n264 = Divide(x=w840, y=w841) -> (x/y=w844:dbl)
                              n265 = Multiply(x=w844, y=100.0) -> (x*y=w842:dbl)
                              n266 = To Unsigned Byte Integer(number=w842) -> (unsigned 8bit integer=w834:u8)
                              n267 = property on="etapa5 barra" class="Slide (strict)"(reference=w835, "Value"=w834) -> ()  [unwired: 1 in, 2 out]
                              n268 = Wait Until Next ms Multiple(millisecond multiple=u32 100) -> ()  [unwired: 1 out]
                            }
                          }
                        }
                      }
                      frame #1 {
                        # "Reactiva busy per seguir amb la seqüència"
                        n269 = flat-sequence {
                          tunnel: w851 -> [w855]
                          tunnel: w850 -> [w853]
                          tunnel: [w853] -> w852
                          tunnel: w852 -> [w856]
                          frame #0 {
                            n270 = property on="busy = T" class="Bool (strict)"(reference=w855, "Value"=TRUE) -> ()  [unwired: 1 in, 2 out]
                          }
                          frame #1 {
                            n271 = Wait (ms)(milliseconds to wait=w856) -> ()  [unwired: 1 out]
                          }
                        }
                      }
                    }
                    n272 = local read "Addresses Cluster"() -> (w789:T1)
                    n273 = To Unsigned Word Integer(number=w794) -> (unsigned 16bit integer=w792:u16[])
                    n274 = To Unsigned Word Integer(number=w795) -> (unsigned 16bit integer=w793:u16[])
                    n275 = flat-sequence {
                      tunnel: w798 -> [w810]
                      tunnel: w791 -> [w812]
                      tunnel: w793 -> [w815]
                      tunnel: [w809] -> w797
                      tunnel: [w808] -> w796
                      tunnel: w792 -> [w814]
                      tunnel: w790 -> [w813]
                      tunnel: w789 -> [w811]
                      frame #0 {
                        # "ACQ DATA analysis and merging"
                        n276 = call "ACQ PostProces1.vi"("ACQ full DATA file path"=w810, "Addresses Cluster"=w811, "Chip ID list 2"=w815, "Chip ID list 1"=w814, "events per file in"=w812, "file sufix num. in"=w813) -> ("events per file out"=w808:u32, "file sufix num. out"=w809:u32)  [unwired: 2 in, 2 out]
                      }
                    }
                  }
                  frame #9 {
                    # "aturar adquisició?"
                    n277 = property on="etapa3 Actual time (ACQ time)" class="DigNum (strict)"(reference=w860) -> ("Value"=w858:u32)  [unwired: 1 in, 2 out]
                    n278 = property on="Stop ACQ" class="Bool (strict)"(reference=w863) -> ("Value"=w862:bool)  [unwired: 1 in, 2 out]
                    n279 = Add(x=w858, y=w859) -> (x+y=w857:u32)
                  }
                }
              }
              n280 = Increment(x=w442) -> (x+1=w441:i32)
              n281 = property on="busy = F" class="Bool (strict)"(reference=w445, "Value"=FALSE) -> ()  [unwired: 1 in, 2 out]
            }
            frame #3 {
              w865 = FALSE ("Value")
              # "3) Finalització a l'adquisició"
              n282 = property on="Stop ACQ button" class="Bool (strict)"(reference=w866, "Visible"=w865, "Value"=w865, "DisabledEnum"=T4."Enabled" ("Disabled")) -> ()  [unwired: 1 in, 2 out]
            }
            frame #4 {
              # "4) Open DATA viewer"
              n283 = local read "ACQ Parameters (cluster)"() -> (w877:T2)
              n284 = property on="ACQ events fets" class="DigNum (strict)"(reference=w880) -> ("Value"=w879:u32)  [unwired: 1 in, 2 out]
              n285 = property on="etapa2 Waiting time (s)" class="DigNum (strict)"(reference=w874) -> ("Value"=w873:u32)  [unwired: 1 in, 2 out]
              n286 = property on="etapa5 Waiting time (s)" class="DigNum (strict)"(reference=w876) -> ("Value"=w872:u32)  [unwired: 1 in, 2 out]
              n287 = property on="Acquisition time (s)" class="DigNum (strict)"(reference=w875) -> ("Value"=w871:u32)  [unwired: 1 in, 2 out]
              n288 = local read "GbReg params"() -> (w884:u8[])
              n289 = property on="HV parameters" class="Clust (strict)"(reference=w885) -> ("Value"=w878:T5)  [unwired: 1 in, 2 out]
              n290 = Index Array "Index Array"(array=w884) -> (element #1=w870:u8, element #2=w869:u8)  [unwired: 2 in]
              n291 = call "Grava_conditionsACQ.vi"("ACQ Parameters (cluster)"=w877, "HV parameters"=w878, "ACQ events fets"=w879, "EQ folder path"=w881, "ACQ folder path"=w882, "EQ loaded?"=w883, "etapa2 Waiting time (s)"=w873, "ACQ anVref low"=w870, "Acquisition time (s)"=w871, "ACQ GbTHLD"=w869, "etapa5 Waiting time (s)"=w872, "HV loops"=w868, "Total ACQ time (s)"=w867) -> ()  [unwired: 7 in]
              n292 = property class="DigNum (strict)"(reference=w880) -> ("Value"=w886:u32)  [unwired: 1 in, 2 out]
              n293 = case shown="..1500000" w886 {
                tunnel: w890 -> [_ w895]
                tunnel: w889 -> [_ w894]
                tunnel: w888 -> [_ w893]
                tunnel: w887 -> [_ w892]
                tunnel: w880 -> [_ w891]
                frame Default {
                }
                frame ..1500000 {
                  n294 = case shown="False" w895 {
                    tunnel: w894 -> [w903 _]
                    tunnel: w893 -> [w902 _]
                    tunnel: w891 -> [w901 _]
                    tunnel: w892 -> [w897 _]
                    frame False {
                      # "No hi ha timeout: obre DATA viewer"
                      n295 = flat-sequence {
                        tunnel: w901 -> [w909]
                        tunnel: w902 -> [w910]
                        tunnel: w903 -> [w911]
                        tunnel: [w911] -> w900
                        tunnel: [w910] -> w899
                        tunnel: [w909] -> w898
                        tunnel: w897 -> [w908]
                        tunnel: [w904] -> w896
                        tunnel: w900 -> [w919]
                        tunnel: w899 -> [w923]
                        tunnel: w898 -> [w922]
                        tunnel: w896 -> [w920]
                        frame #0 {
                          n296 = local read "Chip ID list 1"() -> (w906:u32[])
                          n297 = local read "Chip ID list 2"() -> (w905:u32[])
                          n298 = property on="Operation text" class="Str"(reference=w908, "Value"="Acquiring...\nData viewer open") -> ()  [unwired: 1 in, 2 out]
                          n299 = Build Array (concatenate) "Concatenate"(w906, w905) -> (w904:u32[])
                        }
                        frame #1 {
                          n300 = Strip Path(path=w919) -> (stripped path=w918:path)  [unwired: 1 out]
                          n301 = List Folder(path=w918, pattern="*.dat") -> (filenames=w916:string[])  [unwired: 2 in, 3 out]
                          n302 = Array Size(array=w916) -> (size(s)=w915:i32)
                          n303 = for {
                            N: w915 -> [_]
                            tunnel: w920 -> [w931]
                            tunnel: w919 -> [w933]
                            shift-right: [w935] -> _
                            shift-left: w915 -> [w936]
                            tunnel: [w934] -> w913
                            tunnel: [w932] -> w914
                            tunnel: [w931] -> w912
                            n304 = To Unsigned Long Integer(number=w936) -> (unsigned 32bit integer=w937:u32)
                            n305 = Decrement(x=w936) -> (x-1=w935:i32)
                            n306 = call "Grava_summaryACQ.vi"("sufix number"=w937, "ChipID list"=w931, "ACQ full DATA file path"=w933) -> ("quants events per chip"=w934:u32[], "suffixed file path"=w932:path)  [unwired: 1 in]
                          }
                          n307 = property class="DigNum (strict)"(reference=w922) -> ("Value"=w921:u32)  [unwired: 1 in, 2 out]
                          n308 = case shown="1" w915 {
                            tunnel: w923 -> [_ w930]
                            tunnel: w921 -> [_ w929]
                            tunnel: w914 -> [_ w928]
                            tunnel: w913 -> [_ w926]
                            tunnel: w912 -> [_ w927]
                            frame Default {
                              # "Empty file path\nEmpty ChipID list"
                              # "to choose ACQ file"
                              n309 = call "ACQ_Data_viewer (Module).vi"("ACQ full DATA file path"=path "", "ChipID list"=u32[] []) -> ()  [unwired: 14 in]
                            }
                            frame 1 {
                              # "only one ACQ file"
                              n310 = call "ACQ_Data_viewer (Module).vi"("ACQ full DATA file path"=w928, "ChipID list"=w927, "quants events per chip"=w926, "ID summary"=w930, "ACQ events fets"=w929) -> ()  [unwired: 11 in]
                            }
                          }
                        }
                      }
                    }
                    frame True {
                    }
                  }
                }
              }
            }
          }
        }
      }
    }
    frame True {
      # "connection not working"
      n311 = property on="Error tick" class="Bool (strict)"(reference=w938, "Value"=w939) -> ()  [unwired: 1 in, 2 out]
      n312 = One Button Dialog(message="The connection is NOT WORKING.\n\nCheck the wiring connection and the IP address.") -> ()  [unwired: 1 in, 1 out]
    }
  }
  "Folder path: acquisition reports" <- w1
